vi "HXG2-Main_R2.vi"() -> ()   [LabVIEW 2012]
uses:
  Controls/UI/HXG2_NumDisplayOnlyLarge.ctl
  Controls/UI/HXG2_UI_ControlSetGly.ctl
  Controls/UI/HXG2_UI_ControlSetAir.ctl
  Controls/UI/HXG2_AirENfanRect.ctl
  Controls/UI/HXG2_GlyENfanRect.ctl
  Controls/UI/HXG2_NumDisplayLarge.ctl
  Controls/HXG2_AlarmCluster.ctl
  Controls/UI/HXG2_LED.ctl
  Controls/HXG2_DAQLOOPctrl.ctl
  Modules/Programmer/Data Types/Programmer State.ctl
  Controls/UI/HXG2_NumDisplayOnlySmall.ctl
  Controls/UI/HXG2_MainStateCtrl.ctl
  Controls/UI/HXG2_GralTubeData.ctl
  Controls/UI/HXG2_FinData.ctl
  PID/HXG2_Horizontal PID Control.ctl
  PID/HXG2_Horizontal Reset Control.ctl
  <vilib>/Utility/error.llb/DialogType.ctl
  Modules/Error_Handler/HXG2-Error_Module.ctl
  Modules/Stop/HXG2stop.ctl
  Modules/EnableAirGly/HXG2enable.ctl
  Modules/Timers/HXG2_BlowerPumpl.ctl
  Modules/PID/HXG2pid.ctl
  Modules/Graph_Scales/HXG2_GraphSelections.ctl
  Controls/HXG2_BooleanSelections.ctl
  Modules/BooleanSelections/HXG2boolselec.ctl
  Modules/Save/HXG2save.ctl
  Modules/Save/HXG2saveTimer.ctl
  Modules/AIR-GLY_Clusters/HXG2airglyCluster.ctl
  Controls/HXG2_PIDon-off.ctl
  Modules/DataTransfer/HXG2DataTrans.ctl
  Controls/HXG2_DigitalIn.ctl
  Modules/Programmer/HXG2programmer.ctl
  Modules/Programmer/HXG2programmerUserSelections.ctl
  Modules/Programmer/Data Types/Programmer Execution States.ctl
  Modules/Programmer/HXG2_ProgRefs.ctl
  CondensingVIs/PIDCtrl/HXG2_References.ctl
  <vilib>/Utility/miscctls.llb/LVRowAndColumnTypeDef.ctl
  Controls/HXG2_PIDCluster.ctl
  Controls/HXG2_Aircool-Cascade.ctl
  Controls/HXG2_LiqHeat-Cascade.ctl
  Modules/DAQ/HXG2daq.ctl
  <vilib>/DAQmx/write.llb/DAQmx Write (Digital 1D Bool NChan 1Samp 1Line).vi
panel:
  out "MAIN":bool
  out "DAQ":bool
  in  "HX ID":string="Description #" caption="CHANGE ID OR CLICK TO ACCEPT"
  out "Clear Alarms":bool
  in  "stop":bool
  in  "Master RUN":bool
  out "Main Ctrl":T1
  out "DAQ Control":T2
  out "Event":i32
  out "Main":i32
  out "daq":i32
  in  "Alarm Set Button":bool
  out "error out":errorcluster
  out "Alarm Cluster":T3
  in  "error in (no error)":errorcluster
  out "Programmer":bool
  in  "Tab Control":T5(tab)
  out "dP Inlet":dbl(knob) scale=-10.0..20.0
  out "Pump Pressure (150psi max)":dbl(knob) scale=14.56..50.0
  out "Re Number":dbl format="%#.0f"
  in  "Select Tube OD":u16(ring) items=["3/8\"", "5/16\"", "1/4\"", "3/16\"", "custom"]
  in  "Tube ID (in)":dbl=1.0 min=0.1 max=1.0 format="%#.2f"
  out "Min ACFM 2":dbl format="%#.2f"
  out "Max ACFM 2":dbl format="%#.2f"
  out "HX Pressure In":dbl format="%#.2f psig"
  out "HX dP":dbl format="%#.2f psid"
  out "Pump Pressure":dbl format="%#.2f psig"
  out "Discharge Temp":dbl format="%#.2f °F"
  out "Suction Temp":dbl format="%#.2f °F"
  out "Comp\nSuct SH":dbl format="%#.2f °F"
  out "Comp Suct P psia":dbl(knob) scale=15.0..30.0 scale format="%#.2f"
  in  "Reset Alarm UI":bool
  out "Alarm Present\nLED":bool
  out "Liq Temp °F":T6 min=0.0 max=100.0 format="%#.1f"
  in  "LT PID":bool
  in  "LF PID":bool
  in  "Liq Cluster":T7={"Liq FLOW %"=0.0, "Liq TEMP % "=50.0, "Mdot lbm/hr"=0.0, "TLiq °F"=70.0} caption="Gly Cluster" {"Liq TEMP %" min=0.0 max=100.0 step=1.0 format="%#.1f"; "Liq FLOW %" min=0.0 max=100.0 step=1.0 format="%#.1f"; "TLiq °F" min=40.0 max=180.0 step=1.0 format="%#.1f"; "Mdot lbm/hr" min=0.0 max=1000.0 step=1.0 format="%#.1f"}
  in  "AT PID":bool
  in  "Air Cluster":T8={"Air FLOW %"=30.0, "Air TEMP % "=50.0, "CFMs"=30.0, "Tair  °F"=70.0} {"Air TEMP %" min=0.0 max=100.0 step=1.0 format="%#.1f"; "Air FLOW %" min=0.0 max=100.0 step=1.0 format="%#.1f"; "Tair  °F" min=-5.0 max=100.0 step=1.0 format="%#.1f"; "CFMs" min=0.0 max=200.0 step=1.0 format="%#.1f"}
  in  "Air EN":T9
  out "Air Flow ACFM":T6 min=0.0 max=100.0 format="%#.1f"
  out "Air Temp °F":T6 min=0.0 max=100.0 format="%#.1f"
  in  "LIQ EN":T10
  out "Liq Flow lbm/hr":T11 format="%#.1f"
  in  "Capture Data":bool
  out "Interval Ind":dbl format="%<%H:%M:%S>t"
  out "Duration Ind":dbl format="%<%H:%M:%S>t"
  in  "Duration Ctrl":dbl=15.0 format="%#.1f min"
  in  "Interval Ctrl":dbl=2.0 format="%#.1f s"
  out "File Name":string="Test.tdms"
  out "saving...":bool
  in  "+10":bool
  in  "-10":bool
  in  "Test Point":i32
  in  "AF PID":bool
  out "Pump Pin (psia)":dbl format="%#.2f"
  out "Pump Pout (psia)":dbl format="%#.2f"
  out "UUT dP 0-1.0":dbl format="%.2f inWC"
  out "Liq Htr Well":dbl format="%#.3f °F"
  out "dT Air":dbl format="%#.3f °F"
  out "dT Liq":dbl format="%#.3f °F"
  in  "Sensor":bool
  out "Nozzle dP 2.5inWC":dbl format="%#.3f"
  out "%Bal":string
  out "Max ACFM":dbl format="%#.2f"
  out "Min ACFM":dbl format="%#.2f"
  in  "1\"":bool
  in  "1.25\"":bool
  in  "0.75\"":bool
  in  "1.5\"":bool
  out "Liq q W":dbl format="%#.2f"
  out "Air q W":dbl format="%#.3g"
  out "% Balance":dbl format="%#.1f%"
  out "Air q BTU/hr":dbl format="%#.3g"
  out "Liq q BTU/hr":dbl format="%#.2f"
  out "GlyFlow lbm/hr":dbl format="%#.2f lbm/hr"
  out "LiqCp BTU/lb°F":dbl format="%#.2f"
  out "LiqRho lb/ft³":dbl format="%#.2f"
  out "AirFlow ACFM":dbl format="%#.2f"
  out "AirFlow SCFM":dbl format="%#.2f"
  out "AirCp BTU/lb°F":dbl format="%#.4f"
  out "AirRho lb/ft³":dbl format="%#.4f"
  out "Nozzle °F":dbl format="%#.2f"
  out "UUT °F":dbl format="%#.2f"
  out "Nozzle %RH":dbl format="%#.2f"
  out "UUT %RH":dbl format="%#.2f"
  out "Nozzle dP 5inWC":dbl format="%#.3f"
  out "UUT dP 0-0.1":dbl format="%.3f inWC"
  out "Baro psia":dbl format="%#.2f"
  out "LiqOut Avg °F":dbl format="%#.2f"
  out "LiqIn Avg °F":dbl format="%#.2f"
  out "AirOut Avg °F":dbl format="%#.2f"
  out "AirIn Avg °F":dbl format="%#.2f"
  out "AirOut 8":dbl format="%#.2f"
  out "AirOut 7":dbl format="%#.2f"
  out "AirOut 6":dbl format="%#.2f"
  out "AirOut 4":dbl format="%#.2f"
  out "AirOut 3":dbl format="%#.2f"
  out "AirOut 2":dbl format="%#.2f"
  out "AirOut 1":dbl format="%#.2f"
  in  "AirOut 1 °F":bool
  in  "AirOut 2 °F":bool
  in  "AirOut 3 °F":bool
  in  "AirOut 4 °F":bool
  in  "AirOut 5 °F":bool
  in  "AirOut 6 °F":bool
  in  "AirOut 7 °F":bool
  in  "AirOut 8 °F":bool
  out "AirOut 5":dbl format="%#.2f"
  out "AirIn 4":dbl format="%#.2f"
  out "AirIn 3":dbl format="%#.2f"
  out "AirIn 2":dbl format="%#.2f"
  out "AirIn 1":dbl format="%#.2f"
  in  "AirIn 1 °F":bool
  in  "AirIn 2 °F":bool
  in  "AirIn 3 °F":bool
  in  "AirIn 4 °F":bool
  out "GlyOut 2":dbl format="%#.2f"
  out "GlyOut 1":dbl format="%#.2f"
  in  "LiqOut 1 °F":bool
  in  "LiqOut 2 °F":bool
  out "GlyIn 2":dbl format="%#.2f"
  out "GlyIn 1":dbl format="%#.2f"
  in  "LiqIn 1 °F":bool
  in  "LiqIn 2 °F":bool
  in  "SchedSelect":enum16{"Schedule 1", "Schedule 2", "Schedule 3"}(ring)
  in  "Set Prof 1":bool
  out "Liq Temp":dbl=100.0 format="%#.1f °F"
  out "Mass flow":dbl=100.0 format="%#.1f lbm/hr"
  out "Air Temp":dbl=100.0 format="%#.1f °F"
  out "Air flow":dbl=100.0 format="%#.1f CFM"
  in  "Apply Scales":bool
  in  "Plot Selection":u16[](array[ring]) items=["Liq In Avg", "Liq In 1", "Liq In 2", "Liq Out Avg", "Liq Out 1", "Liq Out 2", "Fltrd Mdot", "Liq Mdot", "Pump 0-250psia", "Pump dP 0-25psid", "UUT 0-100psid", "UUT 0-95psig", "Air In Avg", "Air In 1", "Air In 2", "Air In 3", "Air In 4", "Air Out Avg", "Air Out 1", "Air Out 2", "Air Out 3", "Air Out 4", "Air Out 5", "Air Out 6", "Air Out 7", "Air Out 8", "CFM Nozzle", "CFM HX", "UUT 0-0.1inWC x100", "UUT 0-1inWC x100", "Nozzle 0-5inWC x100", "Nozzle 0-2.5inWC x100", "Pbaro [psia]", "Liq Q (BTU/hr)", "Liq Q (W)", "Air Q (BTU/hr)", "Air Q (W)", "SH (°F)", "SH multiplier", "%Energy Bal", "Liq Re", "AF Ctl Out", "AC Ctl Out", "AH Ctl Out", "LF Ctl Out", "LC Ctl Out", "LH Ctl Out", "Box Btm In (9)", "Box Btm Out (10)", "Box Rt In (11)", "Box Rt Frt (12) ", "Box Top In(13)", "Box Top Out(14)", "Box Lt In (15)", "Box Lt Out (16)", "Evap TR", "Evap TL", "Evap BR", "Evap BL", "Htr Rt", "Htr Top", "Htr Lt", "Htr Btm", "WaterTank"]
  in  "Plot Axis":u32[](array[ring]) items=["1", "2", "3"]
  out "Waveform Chart Out":waveform(dbl)[](graph)
  in  "Max 1":dbl=100.0
  in  "Min 1":dbl
  in  "Max 2":dbl=100.0
  in  "Min 2":dbl
  in  "Max 3":dbl=100.0
  in  "Min 3":dbl
  in  "x-axis length (min)":dbl=1.0
  out "% Balance":dbl format="%#.1f%"
  out "%Bal2":string
  in  "Set Prof 2":bool
  in  "Set Prof 3":bool
  in  "Default":bool
  in  "PID Setup Array":T12
  in  "PID Select":T13(ring)
  in  "Reset PIDs":T14
  in  "Fan TR":bool
  in  "Fan TL":bool
  in  "Fan BL":bool
  in  "Fan BR":bool
  out "Timer":dbl format="%<%H:%M:%S%1u>t"
  in  "HX ID (in)":dbl
  in  "Target Re":dbl
  in  "Liq Tin (°F)":dbl
  out "mdot (lbm/hr)":dbl
  out "mu (lbm/ft*s)":dbl
  out "Cp (BTU/lbm°F)":dbl
  out "Density (lbm/ft³)":dbl
  in  "Repeat Execution:":i32
  in  "Done Stop":bool=TRUE
  in  "Run Programmer":bool
  in  "Load Profile":bool
  in  "Save Profile":bool
  in  "Table":string[][](table) caption="StartProf.prof"
  out "Current Step":i32
  out "Programmer State":T15
  out "AirFlow Stable":bool
  out "AirTemp Stable":bool
  out "LiqFlow Stable":bool
  out "LiqTemp Stable":bool
  out "CFM SP":T16 min=0.0 max=100.0 format="%#.1f"
  out "Tair SP °F":T16 min=0.0 max=100.0 format="%#.1f"
  out "Liq SP lbm/hr":T16 min=0.0 max=100.0 format="%#.1f"
  out "Tliq SP °F":T16 min=0.0 max=100.0 format="%#.1f"
  out "Tliq  °F":T16 min=0.0 max=100.0 format="%#.1f"
  out "Filtered Mdot lbm/hr":T16 min=0.0 max=100.0 format="%#.1f"
  out "Tair  °F":T16 min=0.0 max=100.0 format="%#.1f"
  out "CFM":T16 min=0.0 max=100.0 format="%#.1f"
  out "Ring Text.Text":string
  out "UUTIn 5":dbl format="%#.1f °F"
  out "UUTIn 6":dbl format="%#.1f °F"
  out "UUTIn 7":dbl format="%#.1f °F"
  out "UUTIn 8":dbl format="%#.1f °F"
  out "UUTIn 1":dbl format="%#.1f °F"
  out "UUTIn 2":dbl format="%#.1f °F"
  out "UUTIn 3":dbl format="%#.1f °F"
  out "UUTIn 4":dbl format="%#.1f °F"
  in  "TC 8":string
  in  "TC 7":string
  in  "TC 6":string
  in  "TC 5":string
  in  "TC 4":string
  in  "TC 3":string
  in  "TC 2":string
  in  "TC 1":string
  in  "Prof 3":u16[](array[ring]) items=["Liq In Avg", "Liq In 1", "Liq In 2", "Liq Out Avg", "Liq Out 1", "Liq Out 2", "Fltrd Mdot", "Liq Mdot", "Pump 0-250psia", "Pump dP 0-25psid", "UUT 0-100psid", "UUT 0-95psig", "Air In Avg", "Air In 1", "Air In 2", "Air In 3", "Air In 4", "Air Out Avg", "Air Out 1", "Air Out 2", "Air Out 3", "Air Out 4", "Air Out 5", "Air Out 6", "Air Out 7", "Air Out 8", "CFM Nozzle", "CFM HX", "UUT 0-0.1inWC x100", "UUT 0-1inWC x100", "Nozzle 0-5inWC x100", "Nozzle 0-2.5inWC x100", "Pbaro [psia]", "Liq Q (BTU/hr)", "Liq Q (W)", "Air Q (BTU/hr)", "Air Q (W)", "SH (°F)", "SH multiplier", "%Energy Bal", "Liq Re", "AF Ctl Out", "AC Ctl Out", "AH Ctl Out", "LF Ctl Out", "LC Ctl Out", "LH Ctl Out", "Box Btm In (9)", "Box Btm Out (10)", "Box Rt In (11)", "Box Rt Frt (12) ", "Box Top In(13)", "Box Top Out(14)", "Box Lt In (15)", "Box Lt Out (16)", "Evap TR", "Evap TL", "Evap BR", "Evap BL", "Htr Rt", "Htr Top", "Htr Lt", "Htr Btm", "WaterTank"]
  in  "Prof 2":u16[](array[ring]) items=["Liq In Avg", "Liq In 1", "Liq In 2", "Liq Out Avg", "Liq Out 1", "Liq Out 2", "Fltrd Mdot", "Liq Mdot", "Pump 0-250psia", "Pump dP 0-25psid", "UUT 0-100psid", "UUT 0-95psig", "Air In Avg", "Air In 1", "Air In 2", "Air In 3", "Air In 4", "Air Out Avg", "Air Out 1", "Air Out 2", "Air Out 3", "Air Out 4", "Air Out 5", "Air Out 6", "Air Out 7", "Air Out 8", "CFM Nozzle", "CFM HX", "UUT 0-0.1inWC x100", "UUT 0-1inWC x100", "Nozzle 0-5inWC x100", "Nozzle 0-2.5inWC x100", "Pbaro [psia]", "Liq Q (BTU/hr)", "Liq Q (W)", "Air Q (BTU/hr)", "Air Q (W)", "SH (°F)", "SH multiplier", "%Energy Bal", "Liq Re", "AF Ctl Out", "AC Ctl Out", "AH Ctl Out", "LF Ctl Out", "LC Ctl Out", "LH Ctl Out", "Box Btm In (9)", "Box Btm Out (10)", "Box Rt In (11)", "Box Rt Frt (12) ", "Box Top In(13)", "Box Top Out(14)", "Box Lt In (15)", "Box Lt Out (16)", "Evap TR", "Evap TL", "Evap BR", "Evap BL", "Htr Rt", "Htr Top", "Htr Lt", "Htr Btm", "WaterTank"]
  out "UUTIn 15":dbl format="%#.1f °F"
  out "UUTIn 11":dbl format="%#.1f °F"
  out "UUTIn 10":dbl format="%#.1f °F"
  out "UUTIn 9":dbl format="%#.1f °F"
  out "UUTIn 14":dbl format="%#.1f °F"
  out "UUTIn 13":dbl format="%#.1f °F"
  in  "Accuracy (%of flow)":dbl=0.05
  in  "Repeatability (% of flow)":dbl=0.025
  in  "Select Path":path
  in  "Inlet  Uncert (°F)":dbl=0.09
  in  "Outlet  Uncert (°F)":dbl=0.09
  out "Liquid Power Uncertainty":T17 {"% error T" format="%#.3f"; "% error Power" format="%#.3f"; "% error Mdot" format="%#.3f"; "Power Uncert (BTU/hr)" format="%#.3f"; "Power Uncert (W)" format="%#.3f"}
  out "UUTIn 12":dbl format="%#.1f °F"
  out "UUTIn 16":dbl format="%#.1f °F"
  in  "Prof 1":u16[](array[ring]) items=["Liq In Avg", "Liq In 1", "Liq In 2", "Liq Out Avg", "Liq Out 1", "Liq Out 2", "Fltrd Mdot", "Liq Mdot", "Pump 0-250psia", "Pump dP 0-25psid", "UUT 0-100psid", "UUT 0-95psig", "Air In Avg", "Air In 1", "Air In 2", "Air In 3", "Air In 4", "Air Out Avg", "Air Out 1", "Air Out 2", "Air Out 3", "Air Out 4", "Air Out 5", "Air Out 6", "Air Out 7", "Air Out 8", "CFM Nozzle", "CFM HX", "UUT 0-0.1inWC x100", "UUT 0-1inWC x100", "Nozzle 0-5inWC x100", "Nozzle 0-2.5inWC x100", "Pbaro [psia]", "Liq Q (BTU/hr)", "Liq Q (W)", "Air Q (BTU/hr)", "Air Q (W)", "SH (°F)", "SH multiplier", "%Energy Bal", "Liq Re", "AF Ctl Out", "AC Ctl Out", "AH Ctl Out", "LF Ctl Out", "LC Ctl Out", "LH Ctl Out", "Box Btm In (9)", "Box Btm Out (10)", "Box Rt In (11)", "Box Rt Frt (12) ", "Box Top In(13)", "Box Top Out(14)", "Box Lt In (15)", "Box Lt Out (16)", "Evap TR", "Evap TL", "Evap BR", "Evap BL", "Htr Rt", "Htr Top", "Htr Lt", "Htr Btm", "WaterTank"]
  out "EvapAvg":dbl format="%#.1f °F"
  out "HtrAvg":dbl format="%#.1f °F"
  in  "AirCool Cascade":T18={"PID gains"={"proportional gain (Kc)"=-1.15, "integral time (Ti, min)"=2.44, "derivative time (Td, min)"=0.0}, "output range"={"output high"=100.0, "output low"=10.0}} {"output range"."output low" format="%.2f"; "output range"."output high" format="%.2f"; "PID gains"."derivative time (Td, min)" format="%.3f"; "PID gains"."integral time (Ti, min)" format="%.3f"; "PID gains"."proportional gain (Kc)" format="%.3f"}
  out "Calc Rho (lbm/ft³)":dbl=65.0 format="%#.5f"
  out "T° @ f/meter":dbl=65.0 format="%#.5f"
  out "Cp (BTU/lbm °F)":dbl=65.0 format="%#.4f"
  out "Viscosity (lbm/ft s)":dbl=65.0 format="%#.5f"
  in  "LiqHeat Cascade":T18={"PID gains"={"proportional gain (Kc)"=3.54, "integral time (Ti, min)"=46.25, "derivative time (Td, min)"=0.0}, "output range"={"output high"=100.0, "output low"=0.0}} {"output range"."output low" format="%.2f"; "output range"."output high" format="%.2f"; "PID gains"."derivative time (Td, min)" format="%.3f"; "PID gains"."integral time (Ti, min)" format="%.3f"; "PID gains"."proportional gain (Kc)" format="%.3f"}
  in  "CoilData Tabs":enum32{"General Data", "Fin Data"}(tab)
  in  "General_Tube data":T19 {"Tube vertical spacing (Sf)" format="%#.3f in"; "Tube horizontal spacing (Sr)" format="%#.3f in"; "Tube ID" format="%#.3f in"; "Tube thickness" format="%#.3f in"; "Tube OD" format="%#.3f in"; "Tube test Length (tL)" format="%#.3f in"}
  in  "Fin Data":T20 {"Ext collar length" format="%#.3f in"; "Tubes per plate" format="%#.3f"; "Wire Diameter" format="%#.3f in"; "Fin stretch ratio" format="%#.3f %"; "Fin thickness" format="%#.3f in"; "Fin Width" format="%#.3f in"; "Fin OD" format="%#.3f in"; "Fin contact resistance" format="%#.3f ft² hr °F/BTU"; "Fins per inch (FPI)" format="%#.3f"}
  # "10min"
  # "psia"
  # "dP"
  # "RESET"
  # "On 2.5inWC"
  # "Off 5inWC"
  # "NOZZLES"
  # "TARGETS"
  # "times"
  # "RTDs"
  # "Mass Flow"
  # "GRAPH PROFILES"
  # "1"
  # "2"
  # "3"
  # "Heater Outlet\n(Air into screen)"
  # "Evaporator Outlet\n   (Air into screen)"
  # "Coil Physical Data"
  # "Spine Fin"
  # "Wire Fin"
  # "Plate Fin"
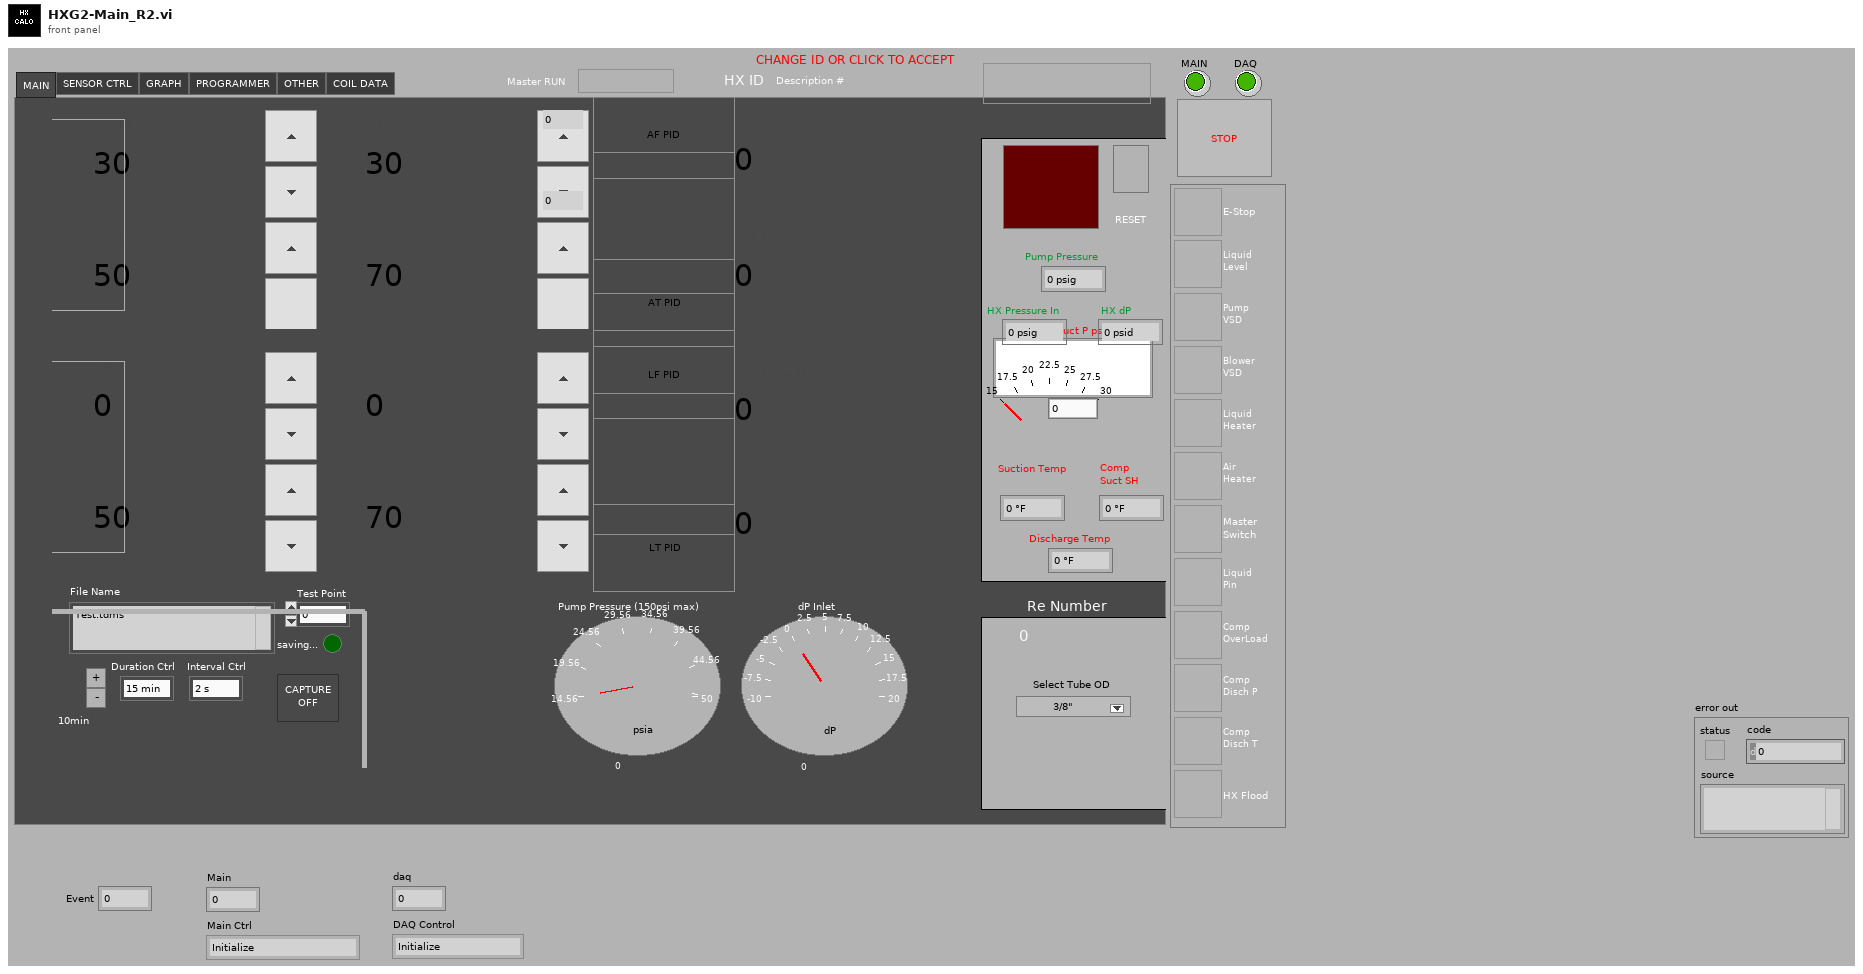
[diagram p1: front panel]
types:
  T1 = typedef "HXG2_MainStateCtrl.ctl" = enum16{"Initialize", "Initialize UI", "DAQ", "Process", "Control", "Write", "Save", "Print", "Graph", "Sequencer", "ERROR", "Exit"}
  T2 = typedef "HXG2_DAQLOOPctrl.ctl" = enum16{"Initialize", "DAQ", "Stop"}
  T3 = typedef "HXG2_AlarmCluster.ctl" = cluster{"E-Stop":T4, "Liquid\nLevel":T4, "Pump\nVSD":T4, "Blower\nVSD":T4, "Liquid\nHeater":T4, "Air\nHeater":T4, "Master\nSwitch":T4, "Liquid\nPin":T4, "Comp\nOverLoad":T4, "Comp\nDisch P":T4, "Comp \nDisch T":T4, "HX Flood":T4}
  T4 = typedef "HXG2_LED.ctl" = bool
  T5 = enum32{"MAIN", "SENSOR CTRL", "GRAPH", "PROGRAMMER", "OTHER", "COIL DATA"}
  T6 = typedef "HXG2_NumDisplayOnlyLarge.ctl" = dbl
  T7 = typedef "HXG2_UI_ControlSetGly.ctl" = cluster{"Liq FLOW %":dbl, "Liq TEMP % ":dbl, "Mdot lbm/hr":dbl, "TLiq °F":dbl}
  T8 = typedef "HXG2_UI_ControlSetAir.ctl" = cluster{"Air FLOW %":dbl, "Air TEMP % ":dbl, "CFMs":dbl, "Tair  °F":dbl}
  T9 = typedef "HXG2_AirENfanRect.ctl" = bool
  T10 = typedef "HXG2_GlyENfanRect.ctl" = bool
  T11 = typedef "HXG2_NumDisplayLarge.ctl" = dbl
  T12 = typedef "HXG2_Horizontal PID Control.ctl" = cluster{"GainsArray":cluster{"Gains 2":cluster{"P":dbl, "I, sec":dbl, "D, sec":dbl}, "Max\nPV":dbl}[], "UL-LL Array":cluster{"UL":dbl, "LL  ":dbl}[]}[]
  T13 = enum16{"AIRFLOW", "AIRCOOL", "AIRHEAT", "LIQFLOW", "LIQCOOL", "LIQHEAT"}
  T14 = typedef "HXG2_Horizontal Reset Control.ctl" = cluster{"AF":bool, "AC":bool, "AH":bool, "LF":bool, "LC":bool, "LH":bool}
  T15 = typedef "Programmer State.ctl" = enum16{"Prepare Next Test Step", "Stopped", "Running", "Stabilizing"}
  T16 = typedef "HXG2_NumDisplayOnlySmall.ctl" = dbl
  T17 = cluster{"Power (BTU/hr)":dbl, "Power Uncert (W)":dbl, "Power Uncert (BTU/hr)":dbl, "% error Mdot":dbl, "% error Power":dbl, "% error T":dbl}
  T18 = cluster{"PID gains":cluster{"proportional gain (Kc)":dbl, "integral time (Ti, min)":dbl, "derivative time (Td, min)":dbl}, "output range":cluster{"output high":dbl, "output low":dbl}}
  T19 = typedef "HXG2_GralTubeData.ctl" = cluster{"Date":string, "Mfr. Name":string, "Tested by":string, "Adv Sys Test#":string, "Model Size/Type":string, "Coil Type":string, "Air flow Direction":enum32{"Radio Selection 1", "Radio Selection 2", "Radio Selection 3"}, "Coil Face Orientation":enum32{"Radio Selection 1", "Radio Selection 2", "Radio Selection 3"}, "Tube Orientation":enum32{"Radio Selection 1", "Radio Selection 2", "Radio Selection 3"}, "Tubes per Bank":dbl, "Number of tube banks":dbl, "Tube test Length (tL)":dbl, "Tube OD":dbl, "Tube thickness":dbl, "Tube ID":dbl, "Tube horizontal spacing (Sr)":dbl, "Tube vertical spacing (Sf)":dbl}
  T20 = typedef "HXG2_FinData.ctl" = cluster{"Fins per inch (FPI)":dbl, "Fin contact resistance":dbl, "Fin OD":dbl, "Fin Width":dbl, "Fin thickness":dbl, "Fin stretch ratio":dbl, "Wire Diameter":dbl, "Tubes per plate":dbl, "Ext collar length":dbl}
  T21 = typedef "HXG2-Error_Module.ctl" = enum16{"Initialize", "Handle", "Report"}
  T22 = typedef "DialogType.ctl" = u16
  T23 = typedef "HXG2stop.ctl" = enum16{"Write", "Pass"}
  T24 = typedef "HXG2enable.ctl" = enum16{"Write Refs", "Write", "Pass"}
  T25 = typedef "HXG2_BlowerPumpl.ctl" = enum16{"Stop", "Start", "Check Time"}
  T26 = typedef "HXG2pid.ctl" = enum16{"Write PID Efforts", "Write PID On-Off", "Pass", "Write PID Refs", "Write PID Gains", "Wrt PID Resets"}
  T27 = typedef "HXG2_GraphSelections.ctl" = enum16{"Load From File", "Plot Selection In", "Plot Axis In", "Graph Scales In", "Apply Scales", "Out"}
  T28 = typedef "HXG2boolselec.ctl" = enum16{"Write", "Pass"}
  T29 = typedef "HXG2_BooleanSelections.ctl" = cluster{"Bool":cluster{"Use GlyIn 1":bool, "Use GlyIn 2":bool, "Use GlyOut 1":bool, "Use GlyOut 2":bool, "Use AirIn 1":bool, "Use AirIn 2":bool, "Use AirIn 3":bool, "Use AirIn 4":bool, "Use AirOut 1":bool, "Use AirOut 2":bool, "Use AirOut 3":bool, "Use AirOut 4":bool, "Use AirOut 5":bool, "Use AirOut 6":bool, "Use AirOut 7":bool, "Use AirOut 8":bool, "0.75in Nozzle":bool, "1.00in Nozzle":bool, "1.25in Nozzle":bool, "1.5in Nozzle":bool, "On 2.5inWC/Off 5inWC":bool, "Fan TR":bool, "Fan TL":bool, "Fan BR":bool, "Fan BL":bool}, "Other":cluster{"Tube ID":dbl}}
  T30 = typedef "HXG2save.ctl" = enum16{"Write", "Pass", "Initialize", "Kill"}
  T31 = typedef "HXG2saveTimer.ctl" = enum16{"EvntStrtDurtn", "EvntStrtInterv", "Stop", "Check", "RegStrtInterv", "Add10Durtn", "Take10Durtn"}
  T32 = typedef "HXG2airglyCluster.ctl" = enum16{"Write", "Pass"}
  T33 = typedef "HXG2_PIDon-off.ctl" = cluster{"AF PID":bool, "AT PID":bool, "LF PID":bool, "LT PID":bool}
  T34 = typedef "HXG2_DigitalIn.ctl" = cluster{"All Digital IN":cluster{"LiqNotlow":bool, "LiqHtrNotOverTemp":bool, "AirHtrNotOverTemp":bool, "BlowerVFD-On":bool, "PumpVFD-On":bool, "CompNotOverloaded":bool, "CompNotOverPdisch":bool, "EMOcleared":bool, "EMOreset":bool, "Master Power Switch":bool, "HX Flood":bool}}
  T35 = typedef "HXG2DataTrans.ctl" = enum16{"Write", "Pass"}
  T36 = typedef "HXG2programmer.ctl" = enum16{"Write Refs", "Write Selec", "Write All", "Pass All", "React", "Write Path"}
  T37 = typedef "HXG2programmerUserSelections.ctl" = cluster{"Run Prog":bool, "Done Stop":bool, "Load Profile":bool, "Save Profile":bool, "Repeat Execution:":i32, "Start Programmer":bool, "Stop Programmer":bool}
  T38 = enum8{"Enabled", "Disabled", "Disabled and Grayed Out"}
  T39 = enum16{"AIRFLOW", "AIRCOOL", "AIRHEAT", "LIQFLOW", "LIQCOOL", "LIQHEAT"}[]
  T40 = enum16{"Schedule 1", "Schedule 2", "Schedule 3"}[]
  T41 = typedef "HXG2_PIDctrlsOUT.ctl" = cluster{"Iteration dT (s)":dbl, "af ctrl effort":dbl, "ac ctrl effort":dbl, "ah ctrl effort":dbl, "lf ctrl effort":dbl, "lc ctrl effort":dbl, "lh ctrl effort":dbl}
  T42 = typedef "HXG2_References.ctl" = cluster{"AF PID ON":refnum<vi>, "AT PID ON":refnum<vi>, "LT PID ON":refnum<vi>, "LF PID ON":refnum<vi>, "Reset Ctrls":refnum<vi>[]}
  T43 = typedef "HXG2_ProgRefs.ctl" = cluster{"Prog. Indicator":refnum<vi>, "Table":refnum<vi>, "Save Button":refnum<vi>, "Duration Ctrl":refnum<vi>, "Run Prog":refnum<vi>}
  T44 = typedef "Programmer Execution States.ctl" = enum16{"Register Steps", "Initialize", "Start Test Sequence", "Register Data", "Execute Programmer", "Set Number of Repetitions", "Get Current Step Index", "Get Time Until Step Ends"}
  T45 = typedef "LVRowAndColumnTypeDef.ctl" = cluster{"Row":i32, "Column":i32}
  T46 = typedef "HXG2_PIDCluster.ctl" = cluster{"PIDon-off ":T33, "PID":T12, "Reset PIDs":T14, "AirCool Cascade":T47, "LiqHeat Cascade":T48}
  T47 = typedef "HXG2_Aircool-Cascade.ctl" = cluster{"PID gains":cluster{"proportional gain (Kc)":dbl, "integral time (Ti, min)":dbl, "derivative time (Td, min)":dbl}, "output range":cluster{"output high":dbl, "output low":dbl}}
  T48 = typedef "HXG2_LiqHeat-Cascade.ctl" = cluster{"PID gains":cluster{"proportional gain (Kc)":dbl, "integral time (Ti, min)":dbl, "derivative time (Td, min)":dbl}, "output range":cluster{"output high":dbl, "output low":dbl}}
  T49 = typedef "HXG2daq.ctl" = enum16{"Write", "Pass", "Initialize", "Stop"}
  T50 = typedef "HXG2_AnalogIn.ctl" = cluster{"ANALOG":cluster{"Liq in 1":dbl, "Liq in 2":dbl, "Liq out 1":dbl, "Liq out 2":dbl, "AIR in 1":dbl, "AIR in 2":dbl, "AIR in 3":dbl, "AIR in 4":dbl, "AIR out 1":dbl, "AIR out 2":dbl, "AIR out 3":dbl, "AIR out 4":dbl, "AIR out 5":dbl, "AIR out 6":dbl, "AIR out 7":dbl, "AIR out 8":dbl, "RH in Temp":dbl, "RH in":dbl, "RHout Temp":dbl, "RH out":dbl, "Comp Suct P":dbl, "Pabs nozzle":dbl, "Nozzle dp 0-5":dbl, "UUT dp 0-pt1":dbl, "Nozzle dP 0-2.5":dbl, "Pmp  0-250psia":dbl, "UUT  0-100psid":dbl, "UUT 0-50psia":dbl, "TC in 1":dbl, "TC in 2":dbl, "TC in 3":dbl, "TC in 4":dbl, "TC in 5":dbl, "TC in 6":dbl, "TC in 7":dbl, "TC in 8":dbl, "TC in 9":dbl, "TC in 10":dbl, "TC in 11":dbl, "TC in 12":dbl, "TC in 13":dbl, "TC in 14":dbl, "TC in 15":dbl, "TC in 16":dbl, "Liq Mdot":dbl, "UUT dP 0-1":dbl, "Pump dP 0-25":dbl}, "TCsComp":cluster{"CompSuct °F  ":dbl, "CompDisch °F":dbl, "LiqHtrWell °F":dbl}}
  T51 = cluster{"Excel/Elapsed t":dbl[], "Digital In":T34, "Analog In":T50}
  T52 = typedef "HXG2_AirGly-Cluster.ctl" = cluster{"Air Cluster":T8, "Liq Cluster":T7}
  T53 = cluster{"Airflow (CFM)":dbl, "Air Temp (°F)":dbl, "Glycol Flow (lbm/hr)":dbl, "Glycol Temp(°F)":dbl}
  T54 = typedef "HXG2_Calculated.ctl" = cluster{"Means":cluster{"Liq In Avg":dbl, "Liq Out Avg":dbl, "Air In Avg":dbl, "Air Out Avg":dbl, "%Energy Bal":dbl, "Air Evap Avg":dbl, "Air Htr Avg":dbl, "Air Q low":bool}, "Air":cluster{"Min ACFM":dbl, "Max ACFM":dbl, "CFM nozzle":dbl, "CFM HX":dbl, "Air Q (Btu/hr)":dbl, "Air Q (W)":dbl, "Air Cp (Btu/lb)":dbl, "Air rho (lbm/ft³)":dbl}, "Liq":cluster{"Liq rho (lbm/ft³)":dbl, "Liq Cp (Btu/lb)":dbl, "Liq Q (Btu/hr)":dbl, "Liq Q (W)":dbl, "Liq mu (lbm/ft sec)":dbl, "Liq Conc (%)":dbl, "Tube ID (in)":dbl, "Liq Re":dbl, "Mdot Sensor °F":dbl, "Fltrd Mdot (lbm/hr)":dbl}, "SuperHeat":cluster{"SuperHeat °F":dbl, "Multiplier":dbl}, "dT":cluster{"Air dT °F":dbl, "Liq dT °F":dbl}}
  T55 = typedef "HXG2_MaxConstants.ctl" = cluster{"IN":cluster{"all Digital":refnum<k21>, "all DAQ":refnum<k21>, "Analog 480panel":refnum<k21>, "Freq_Mdot":refnum<k21>}, "OUT":cluster{"DIGITAL":cluster{"all DIGITAL":refnum<k21>}, "allANALOG":cluster{"all ANALOG":refnum<k21>}}}
  T56 = cluster{"Components Stable?[0]":bool, "Components Stable?[1]":bool, "Components Stable?[2]":bool, "Components Stable?[3]":bool}
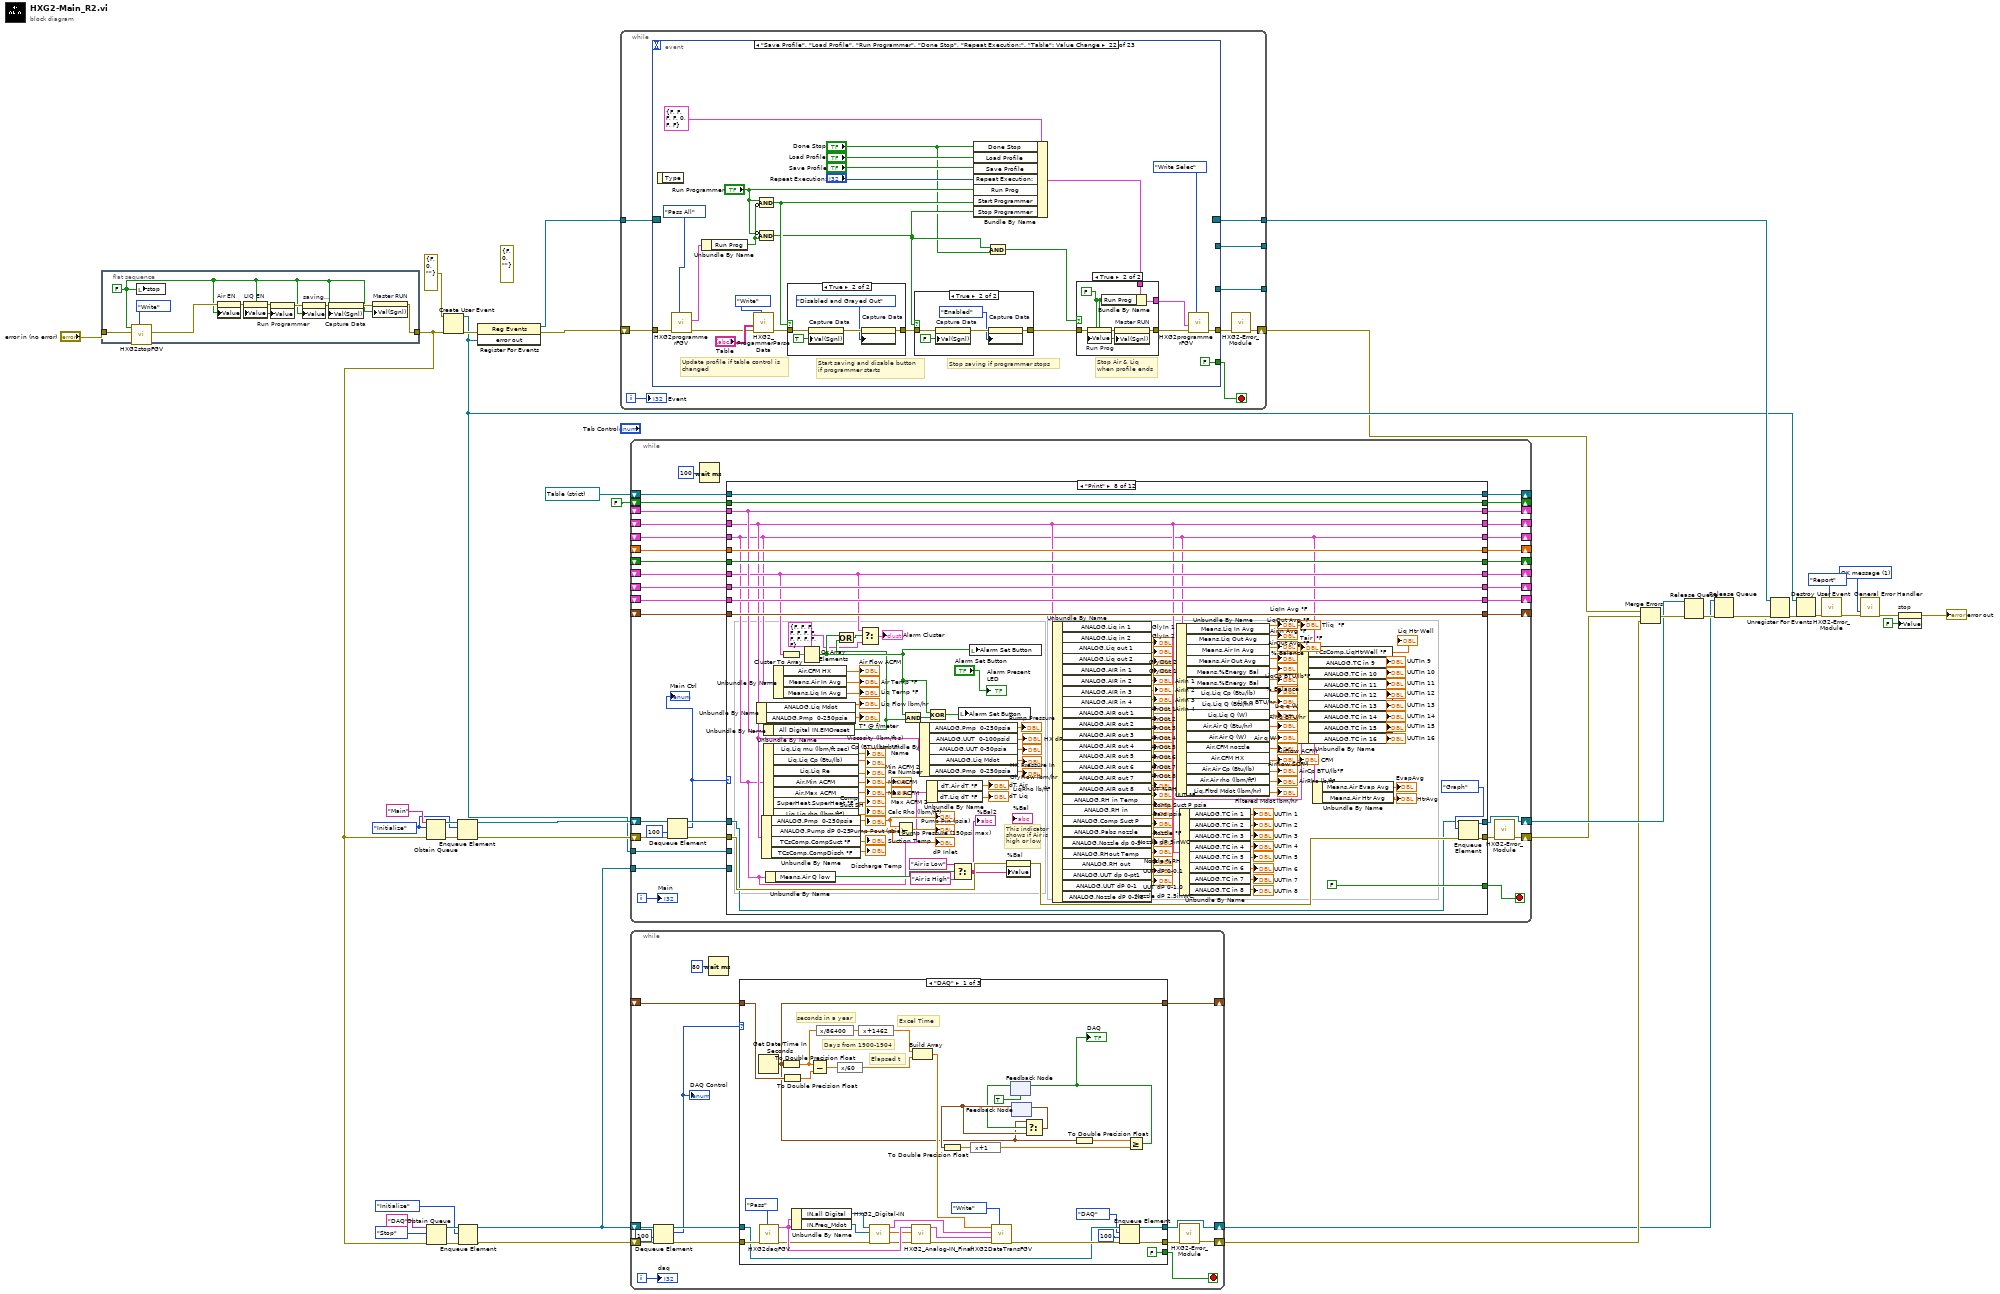
[diagram p0: block diagram]
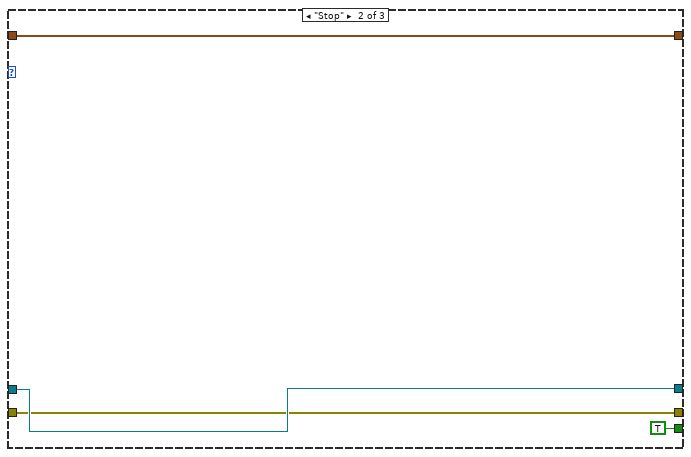
[diagram p2: hidden frame]
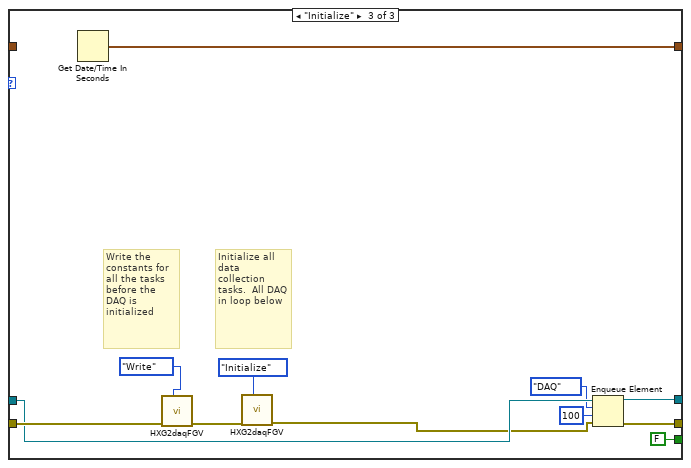
[diagram p3: hidden frame]
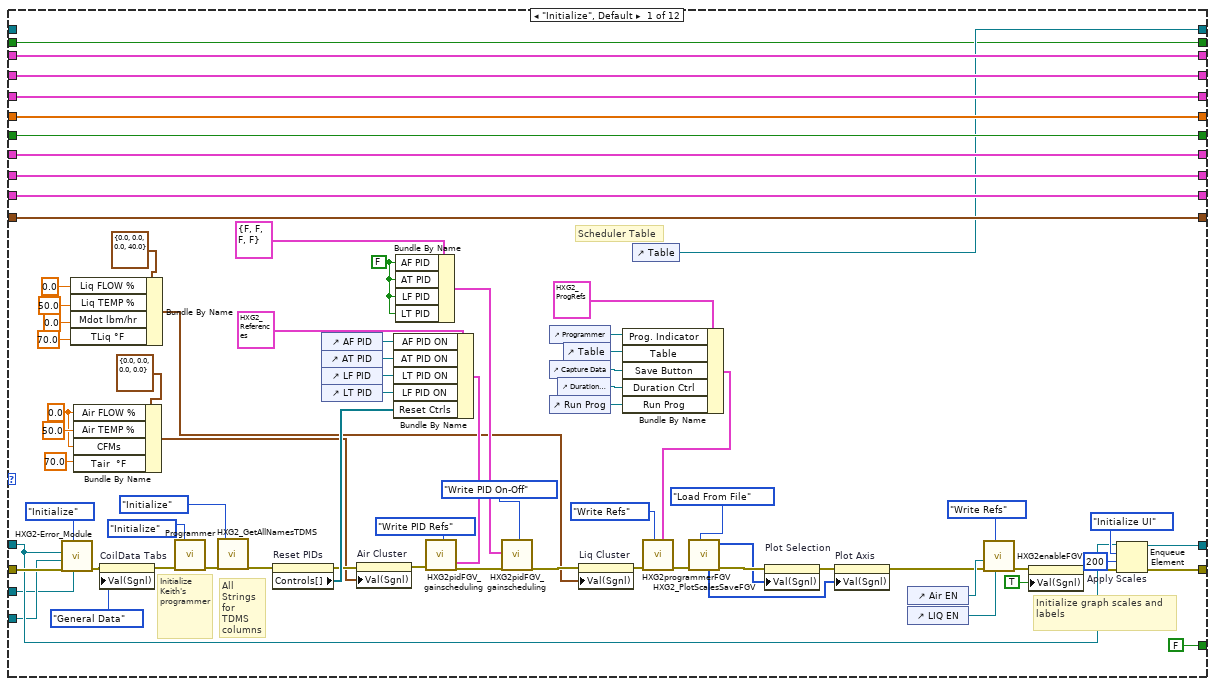
[diagram p4: hidden frame]
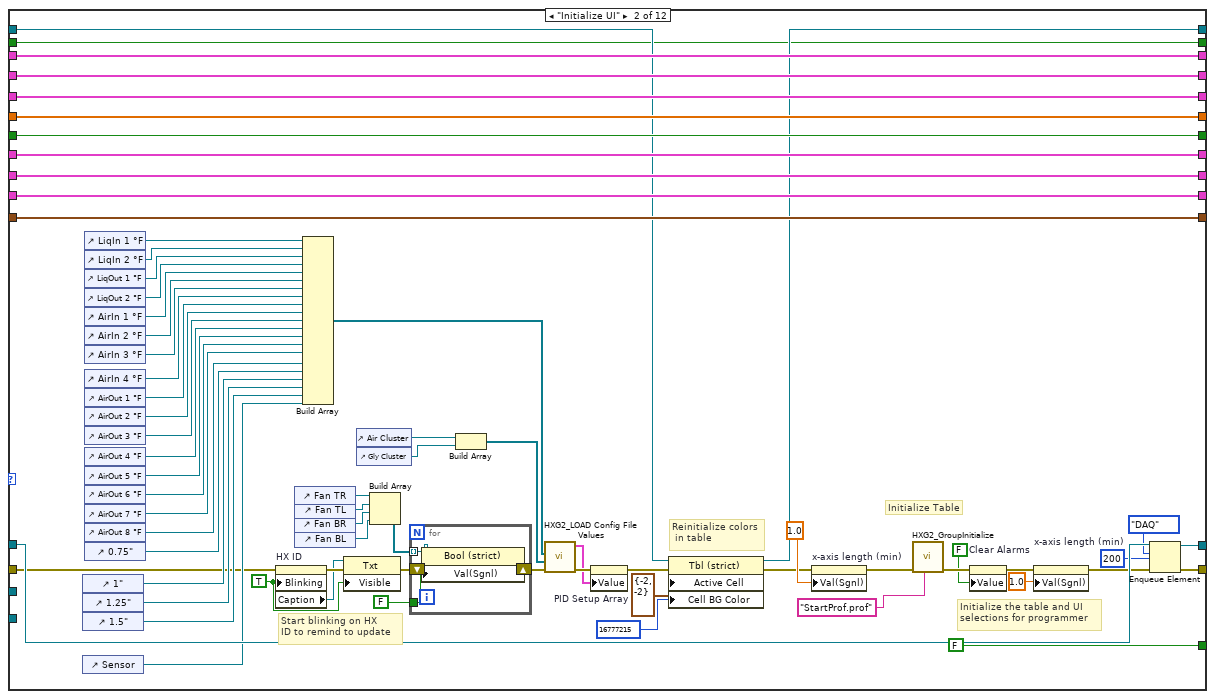
[diagram p5: hidden frame]
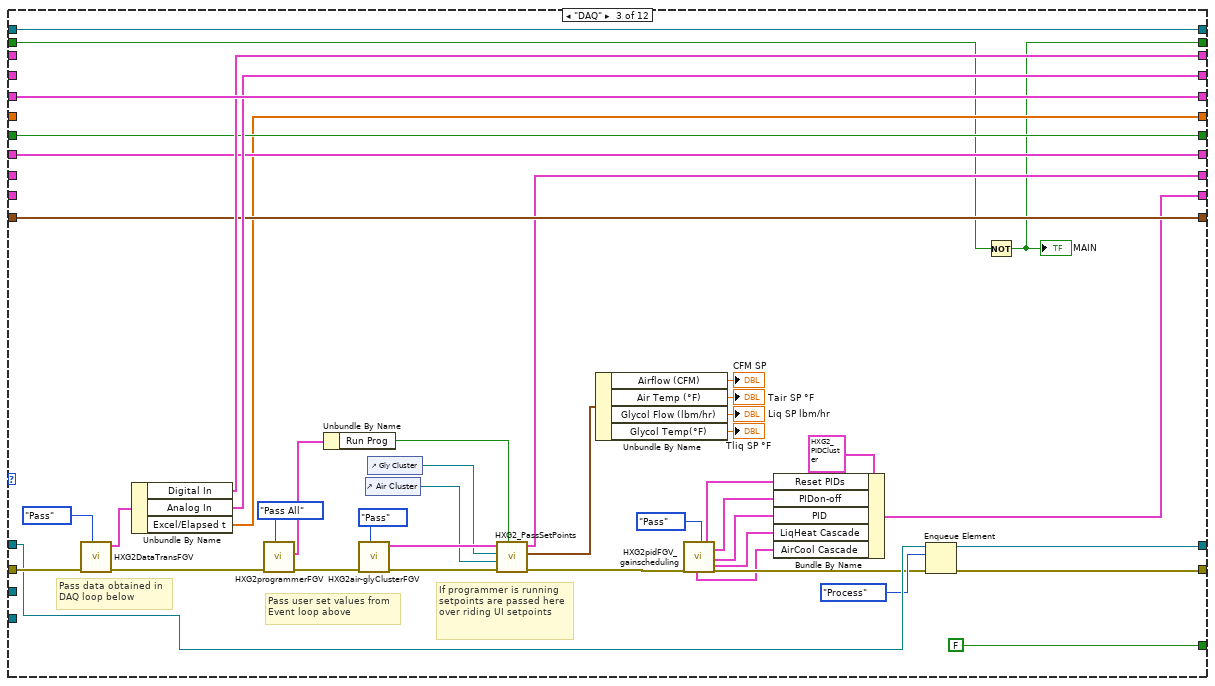
[diagram p6: hidden frame]
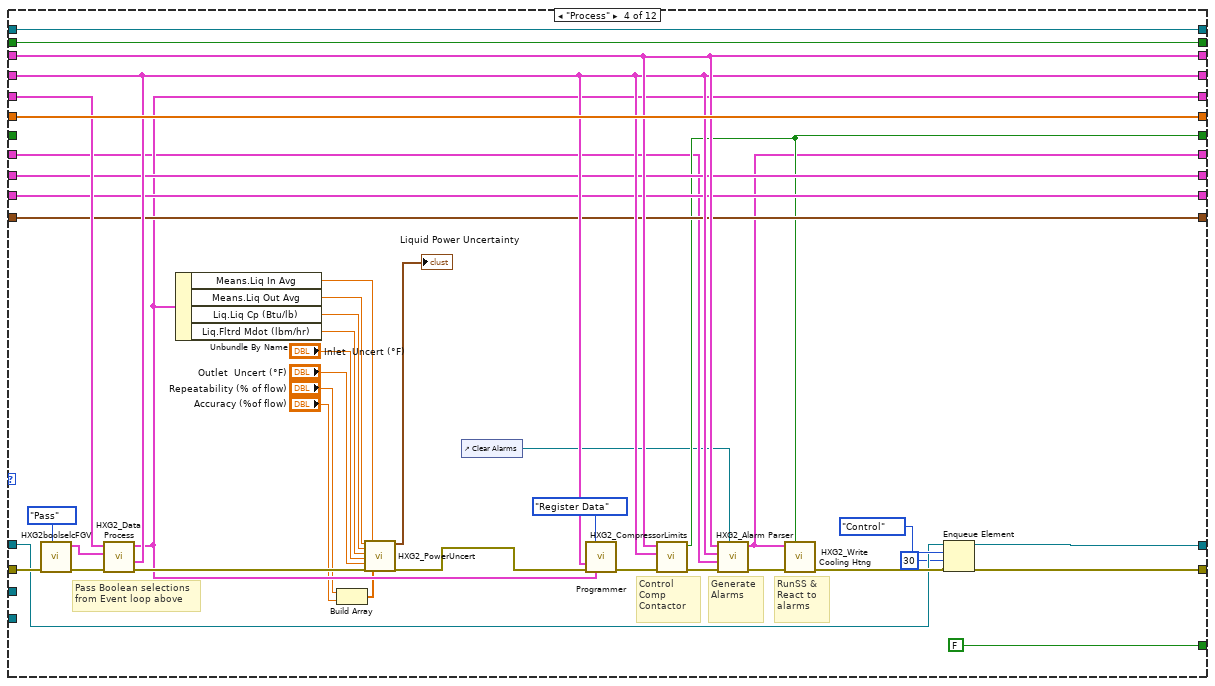
[diagram p7: hidden frame]
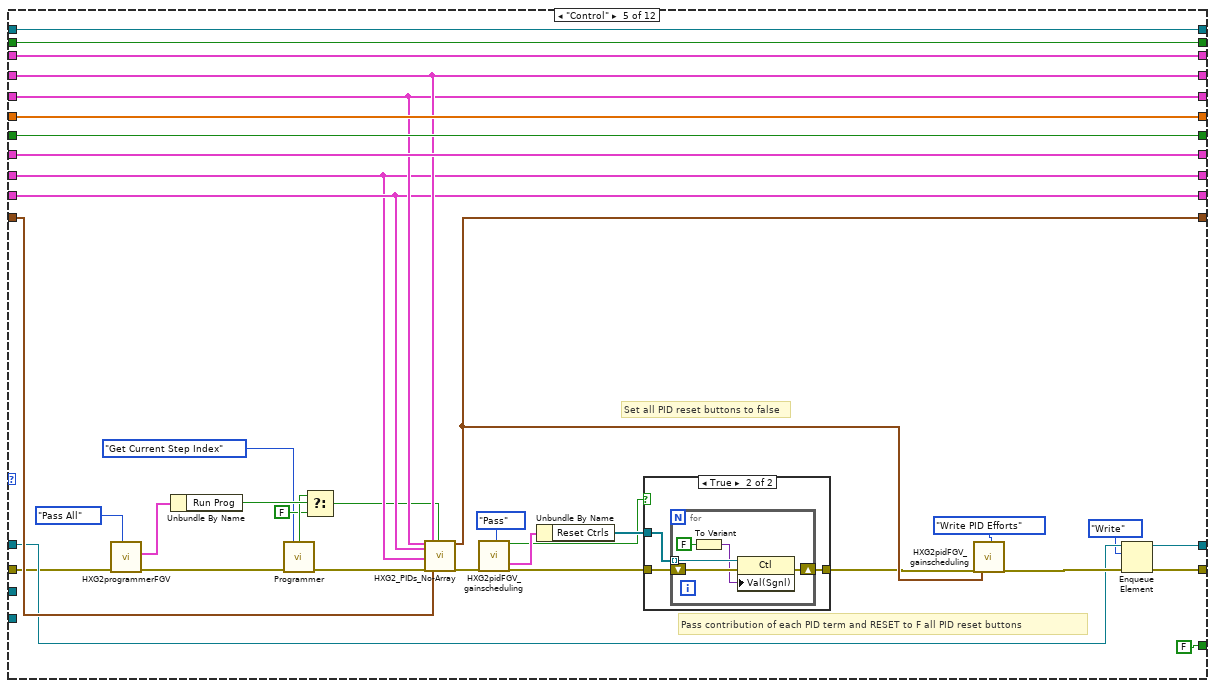
[diagram p8: hidden frame]
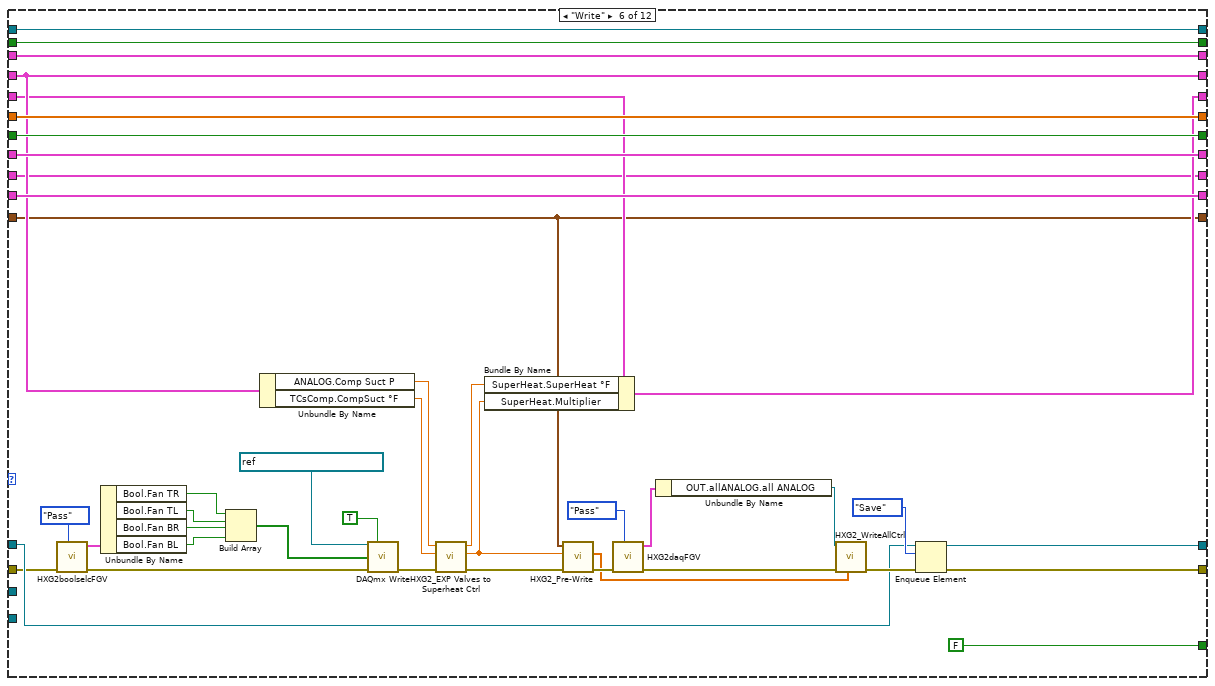
[diagram p10: hidden frame]
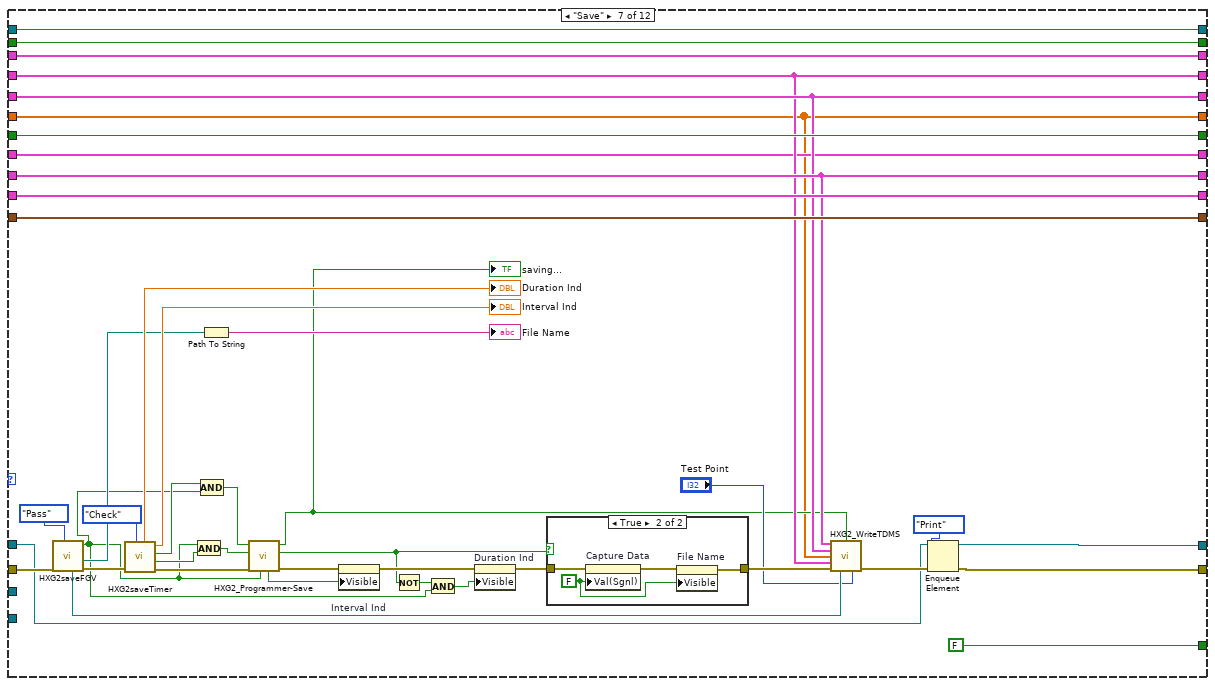
[diagram p11: hidden frame]
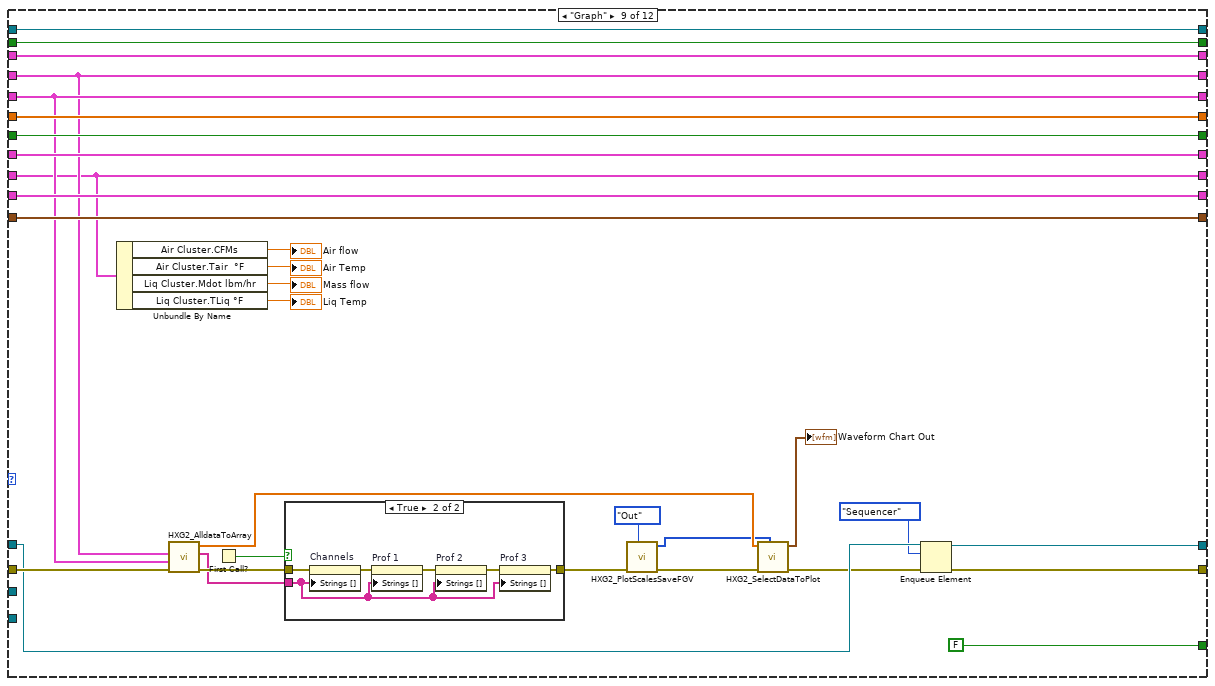
[diagram p13: hidden frame]
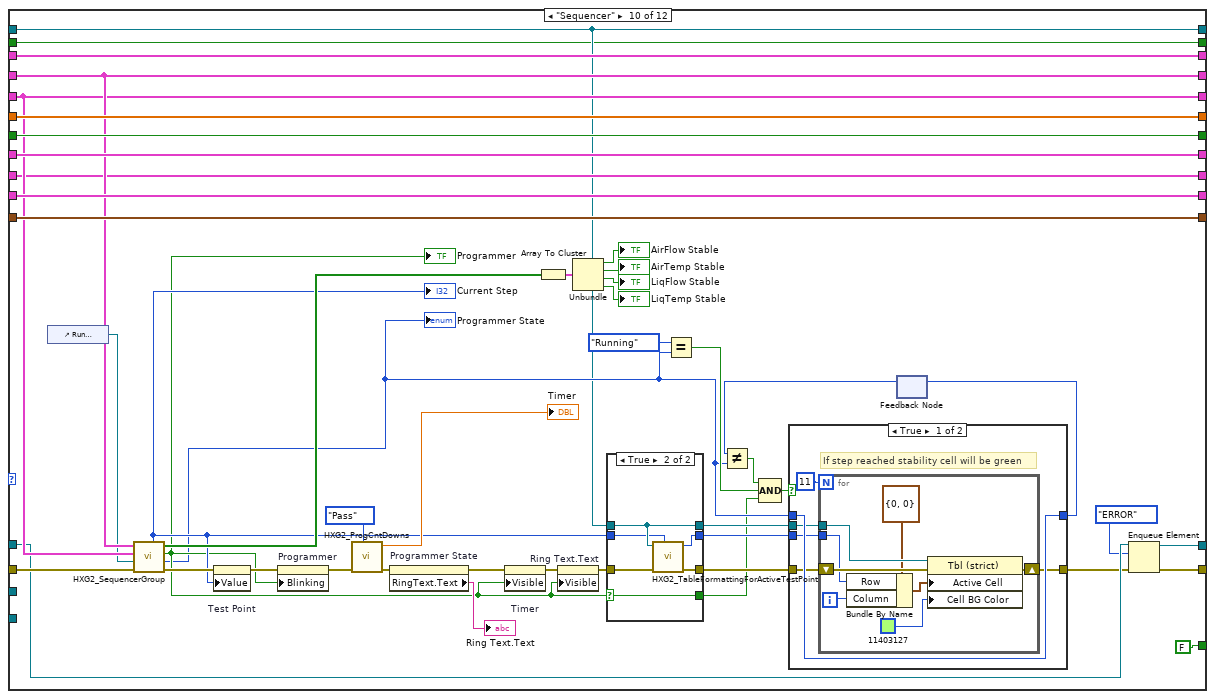
[diagram p15: hidden frame]
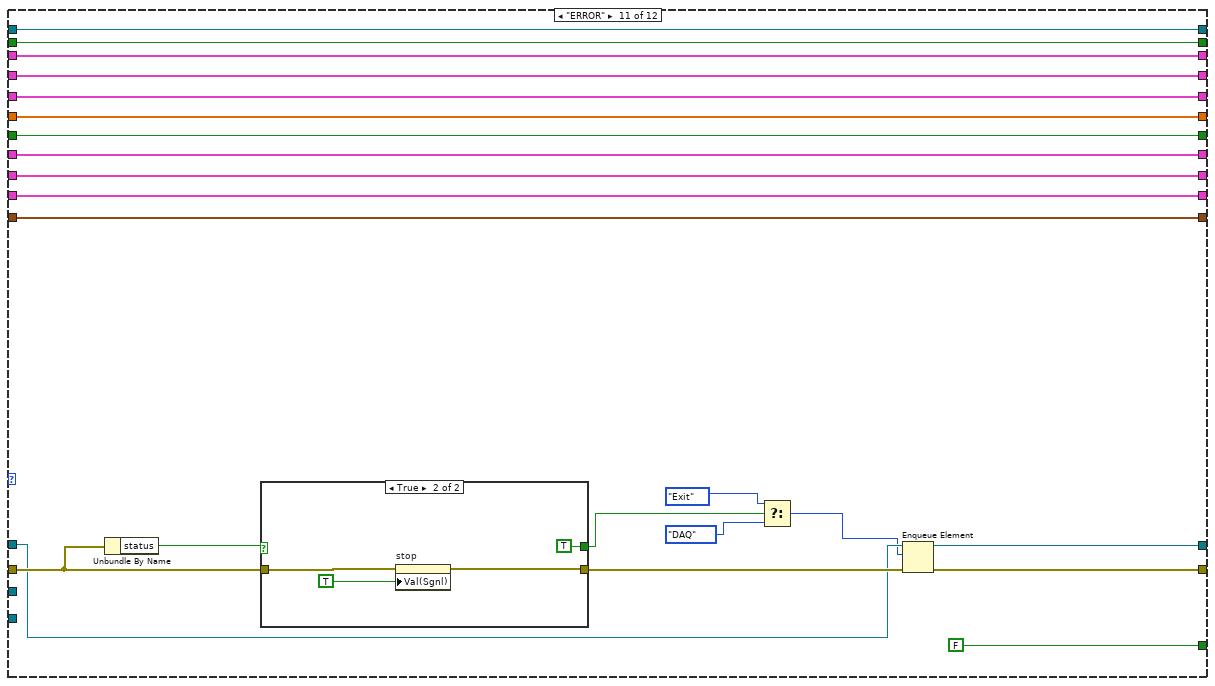
[diagram p18: hidden frame]
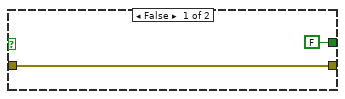
[diagram p19: hidden frame]
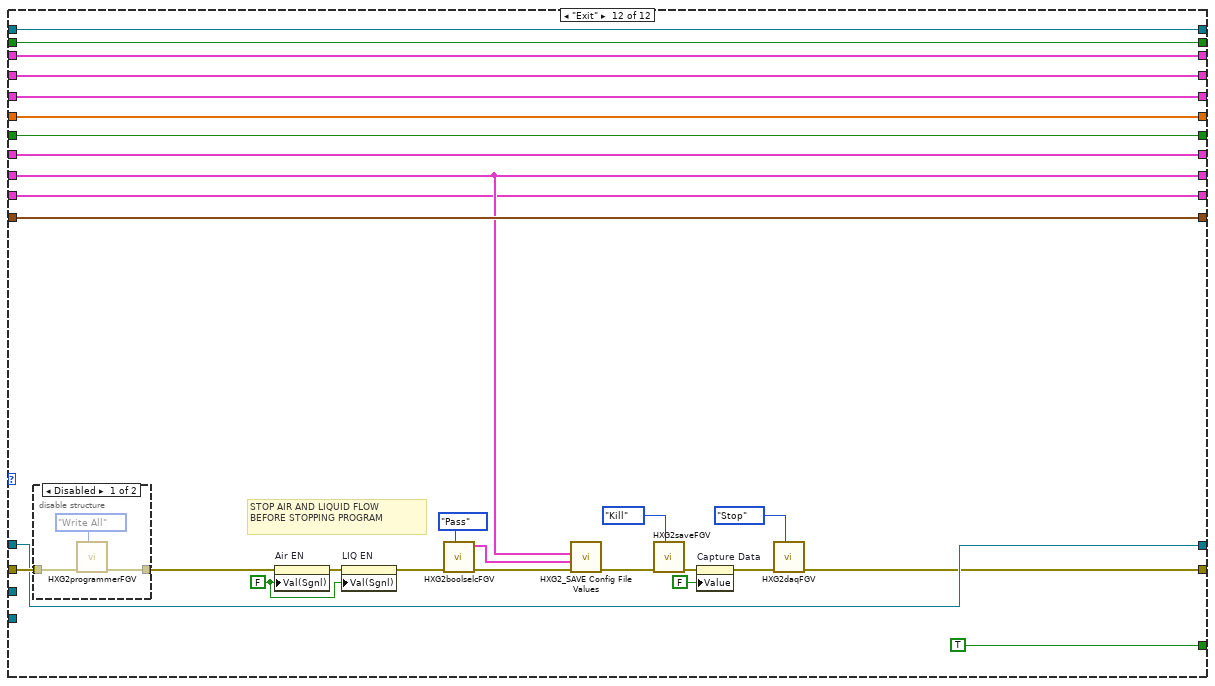
[diagram p20: hidden frame]
diagram:
  (unwired) errorcluster {"status"=FALSE, "code"=0, "source"=""} ("error out")
  w24 = HXG2_MainStateCtrl."Initialize" ("Main State Ctrl")
  w39 = T22 1 items=["no dialog", "OK message", "continue or stop message", "OK message + warnings", "continue/stop + warnings"] ("type of dialog (OK msg:1)")
  n1 = flat-sequence {
    tunnel: [w41] -> w19
    tunnel: "error in (no error)" -> [w49]
    frame #0 {
      w40 = FALSE ("stop")
      n2 = call "HXG2stopFGV.vi"("stopFGV"=HXG2stop."Write", "error in (no error)"=w49, "STOP"=w40) -> ("error out"=w47:errorcluster)  [unwired: 7 in, 1 out]
      n3 = local write "stop"(w40) -> ()
      n4 = property on="Air EN" class="Bool (strict)"(error in=w47, "Value"=w40) -> (error out=w46:errorcluster)  [unwired: 1 in, 1 out]
      n5 = property on="LIQ EN" class="Bool (strict)"(error in=w46, "Value"=w40) -> (error out=w45:errorcluster)  [unwired: 1 in, 1 out]
      n6 = property on="Run Programmer" class="Bool (strict)"(error in=w45, "Value"=w40) -> (error out=w44:errorcluster)  [unwired: 1 in, 1 out]
      n7 = property on="saving..." class="Bool (strict)"(error in=w44, "Value"=w40) -> (error out=w43:errorcluster)  [unwired: 1 in, 1 out]
      n8 = property on="Capture Data" class="Bool (strict)"(error in=w43, "Val(Sgnl)"=w40) -> (error out=w42:errorcluster)  [unwired: 1 in, 1 out]
      n9 = property on="Master RUN" class="Bool (strict)"(error in=w42, "Val(Sgnl)"=w40) -> (error out=w41:errorcluster)  [unwired: 1 in, 1 out]
    }
  }
  n10 = Obtain Queue(name (unnamed)="Main", element data type=w24, error in (no error)=w19) -> (queue out=w29:refnum<queue>, error out=w30:errorcluster)  [unwired: 2 in, 1 out]
  n11 = Obtain Queue(name (unnamed)="DAQ", element data type=HXG2_DAQLOOPctrl."Stop" ("DAQ Control"), error in (no error)=w19) -> (queue out=w34:refnum<queue>, error out=w33:errorcluster)  [unwired: 2 in, 1 out]
  n12 = Create User Event(user event datatype=errorcluster {"status"=FALSE, "code"=0, "source"=""} ("error out"), error in=w19) -> (user event=w12:refnum<user-event>, error out=w18:errorcluster)
  n13 = Enqueue Element(queue=w29, element=w24, error in (no error)=w30) -> (queue out=w26:refnum<queue>, error out=w27:errorcluster)  [unwired: 1 in, 1 out]
  n14 = Enqueue Element(queue=w34, element=HXG2_DAQLOOPctrl."Initialize" ("DAQ Control"), error in (no error)=w33) -> (queue out=w22:refnum<queue>, error out=w32:errorcluster)  [unwired: 1 in, 1 out]
  n15 = register-events(error in=w18, w12) -> (reference out=w16:refnum<event-registration>, error out=w17:errorcluster)  [unwired: 1 in]
  n16 = while {
    shift-right: [w54] -> w8
    shift-left: w17 -> [w58]
    tunnel: [w56] -> _
    tunnel: [w55] -> _
    tunnel: w16 -> [w51]
    tunnel: [w50] -> w13
    i -> [w57]
    stop <- w52 stop-if-true
    n17 = event shown="[21] \"Save Profile\", \"Load Profile\", \"Run Programmer\", \"Done Stop\", \"Repeat Execution:\", \"Table\": Value Change" {
      selector: w51 -> [_ _ _ _ _ _ _ _ _ _ _ _ _ _ _ _ _ _ _ _ _ _ _]
      dyn-events: [_ _ _ _ _ _ _ _ _ _ _ _ _ _ _ _ _ _ _ _ _ _ _] -> w50
      timeout: _ -> [_ _ _ _ _ _ _ _ _ _ _ _ _ _ _ _ _ _ _ _ _ _ _]
      tunnel: [FALSE FALSE ("stop") _ _ _ FALSE ("stop") "stop" TRUE ("stop") FALSE ("stop") _ FALSE _ _ FALSE ("stop") FALSE ("stop") _ _ _ FALSE ("stop") FALSE ("stop") FALSE ("stop") FALSE ("stop") _] -> w52
      tunnel: w58 -> [w59 w75 w155 w180 w181 w210 w219 w234 w244 w288 w296 w349 w352 w361 w381 w384 w393 w405 w414 w438 w498 w526 w567]
      tunnel: [w59 w77 w142 w179 w189 w204 w221 w234 w249 w287 w302 w345 w351 w354 w380 w386 w392 w404 w406 w435 w497 w533 w570] -> w53
      tunnel: [_ _ _ _ _ _ w227 _ _ _ _ _ _ _ _ _ _ _ _ _ _ _ _] -> w56
      tunnel: [_ _ _ _ _ _ w220 _ _ _ _ _ _ _ _ _ _ _ _ _ _ _ _] -> w55
      event Timeout {
        n18 = event-data() -> ()  [unwired: 1 in, 2 out]
      }
      event Value Change {
        w61 = T14 {"AF"=FALSE, "AC"=FALSE, "AH"=FALSE, "LF"=FALSE, "LC"=FALSE, "LH"=FALSE}  # Reset PIDs
        # "-SWITCH FROM PID TO MANUAL OPERATION WHEN AIR AND LIQ ARE\nSTOPPED\n- Start timers to detect drive malfunction when AIR and LIQ are ENABLED"
        n19 = event-data() -> ()  [unwired: 1 in, 2 out]
        n20 = call "HXG2enableFGV.vi"("ENABLE Ctrl"=HXG2enable."Pass", "error in (no error)"=w75) -> ("error out"=w74:errorcluster, "Air-Liq Out"=w72:bool[])  [unwired: 7 in, 1 out]
        n21 = control-ref of="AF PID"() -> (w83:refnum<vi>)
        n22 = control-ref of="AT PID"() -> (w82:refnum<vi>)
        n23 = control-ref of="LF PID"() -> (w80:refnum<vi>)
        n24 = control-ref of="LT PID"() -> (w79:refnum<vi>)
        n25 = Index Array(array=w72, index #1=0 ("index"), index #2=1 ("index")) -> (element #1=w68:bool, element #2=w69:bool)
        n26 = Compound Arithmetic op=AND("Air EN", invert w68) -> (w66:T9)
        n27 = Compound Arithmetic op=AND("LIQ EN", invert w69) -> (w67:T10)
        n28 = Build Array(w83, w82) -> (w81:refnum<vi>[])
        n29 = Build Array(w80, w79) -> (w78:refnum<vi>[])
        n30 = call "HXG2enableFGV.vi"("ENABLE Ctrl"=HXG2enable."Write" ("ENABLE"), "error in (no error)"=w74, "LIQ EN"="LIQ EN", "Air EN"="Air EN") -> ("error out"=w84:errorcluster)  [unwired: 5 in, 2 out]
        n31 = case shown="True" "LIQ EN" {
          tunnel: w84 -> [w123 w134]
          tunnel: [w121 w135] -> w63
          tunnel: w78 -> [_ w132]
          tunnel: w67 -> [w120 _]
          tunnel: w61 -> [w119 _]
          frame True {
            n32 = call "HXG2_Timing Module Pump.vi"("Timer Command"=HXG2_BlowerPumpl."Start", "error in (no error)"=w123) -> ("error out"=w122:errorcluster)  [unwired: 7 in, 2 out]
            n33 = case shown="True" w120 {
              selector: w120 -> [_ w126]
              tunnel: w122 -> [w125 w130]
              tunnel: [w125 w129] -> w121
              tunnel: w119 -> [_ w128]
              frame False {
              }
              frame True {
                n34 = Bundle By Name(cluster=w128, "LF"=w126, "LC"=w126, "LH"=w126) -> (w127:T14)
                n35 = call "HXG2pidFGV_gainscheduling.vi"("error in (no error)"=w130, "Reset PIDs"=w127, "PIDfgvCtrl"=HXG2pid."Wrt PID Resets") -> ("error out"=w129:errorcluster)  [unwired: 8 in, 8 out]
              }
            }
          }
          frame False {
            n36 = for {
              shift-right: [w139] -> w133
              shift-left: w134 -> [w140]
              tunnel: w132 -> [w138] mode=indexing
              n37 = property class="Bool (strict)"(reference=w138, error in=w140, "Val(Sgnl)"=FALSE ("stop")) -> (error out=w139:errorcluster)  [unwired: 1 out]
            }
            n38 = call "HXG2_Timing Module Pump.vi"("Timer Command"=HXG2_BlowerPumpl."Stop", "error in (no error)"=w133) -> ("error out"=w135:errorcluster)  [unwired: 7 in, 2 out]
          }
        }
        n39 = case shown="True" "Air EN" {
          tunnel: w63 -> [w97 w112]
          tunnel: [w96 w113] -> w62
          tunnel: w81 -> [_ w110]
          tunnel: w66 -> [w94 _]
          tunnel: w61 -> [w93 _]
          frame True {
            n40 = call "HXG2_Timing Module Blower.vi"("Timer Command"=HXG2_BlowerPumpl."Start", "error in (no error)"=w97) -> ("error out"=w95:errorcluster)  [unwired: 7 in, 2 out]
            n41 = case shown="True" w94 {
              selector: w94 -> [_ w100]
              tunnel: [w99 w104] -> w96
              tunnel: w95 -> [w99 w108]
              tunnel: w93 -> [_ w101]
              frame False {
              }
              frame True {
                w106 = TRUE ("Blinking")
                n42 = Bundle By Name(cluster=w101, "AF"=w100, "AC"=w100, "AH"=w100) -> (w102:T14)
                n43 = call "HXG2pidFGV_gainscheduling.vi"("error in (no error)"=w108, "Reset PIDs"=w102, "PIDfgvCtrl"=HXG2pid."Wrt PID Resets") -> ("error out"=w103:errorcluster)  [unwired: 8 in, 8 out]
                n44 = property on="HX ID" class="Str"(error in=w103, "Blinking"=w106) -> (error out=w107:errorcluster, "Caption"=w105:refnum<vi>)  [unwired: 1 in, 1 out]
                n45 = property class="Txt"(reference=w105, error in=w107, "Visible"=w106) -> (error out=w104:errorcluster)  [unwired: 1 out]
              }
            }
          }
          frame False {
            n46 = for {
              shift-right: [w117] -> w111
              shift-left: w112 -> [w118]
              tunnel: w110 -> [w116] mode=indexing
              n47 = property class="Bool (strict)"(reference=w116, error in=w118, "Val(Sgnl)"=FALSE ("stop")) -> (error out=w117:errorcluster)  [unwired: 1 out]
            }
            n48 = call "HXG2_Timing Module Blower.vi"("Timer Command"=HXG2_BlowerPumpl."Stop", "error in (no error)"=w111) -> ("error out"=w113:errorcluster)  [unwired: 7 in, 2 out]
          }
        }
        n49 = Or(x="Air EN", y="LIQ EN") -> (x .or. y?=w76:T9)
        n50 = case shown="False" w76 {
          selector: w76 -> [_ w90]
          tunnel: w62 -> [w89 w92]
          tunnel: [w88 w91] -> w77
          frame True {
            n51 = property on="Master RUN" class="Bool (strict)"(error in=w89, "Value"=TRUE ("Master RUN")) -> (error out=w88:errorcluster)  [unwired: 1 in, 1 out]
          }
          frame False {
            n52 = property on="Master RUN" class="Bool (strict)"(error in=w92, "Value"=w90) -> (error out=w91:errorcluster)  [unwired: 1 in, 1 out]
          }
        }
      }
      event "Set Prof 1", "Set Prof 2", "Set Prof 3": Value Change {
        w149 = u16[] [1, 43, 44, 7, 12, 40, 41, 27, 26, 37] items=["none", "Liq In Avg", "Liq In 1", "Liq In 2", "Liq Out Avg", "Liq Out 1", "Liq Out 2", "Fltrd Mdot", "Liq Mdot", "Liq T° f/mtr", "Liq dP 0-25psi", "Liq Pin 0-100psi", "Air In Avg", "Air In 1", "Air In 2", "Air In 3", "Air In 4", "Air Out Avg", "Air Out 1", "Air Out 2", "Air Out 3", "Air Out 4", "Air Out 5", "Air Out 6", "Air Out 7", "Air Out 8", "CFM Nozzle", "CFM HX", "UUT 0-0.1inWC x100", "Chmb 0-5inWC x100", "Chmb 0-2.5inWC x100", "Liq Q (BTU/hr)", "Liq Q (W)", "Air Q (BTU/hr)", "Air Q (W)", "SH (°F)", "SH multiplier", "%Energy Bal", "Liq Re", "AF Ctl Out", "AC Ctl Out", "AH Ctl Out", "LF Ctl Out", "LC Ctl Out", "LH Ctl Out"] ("Plot Selection")
        # "GRAPH PROFILES"
        n53 = event-data() -> ()  [unwired: 1 in, 5 out]
        n54 = case shown="True" "Set Prof 1" {
          tunnel: w155 -> [w173 w174]
          tunnel: [w173 w176] -> w154
          frame False {
          }
          frame True {
            n55 = property on="Plot Selection" class="Arr (strict)"(error in=w174, "Value"="Prof 1") -> (error out=w176:errorcluster)  [unwired: 1 in, 1 out]
          }
        }
        n56 = control-ref of="Set Prof 1"() -> (w147:refnum<vi>)
        n57 = control-ref of="Set Prof 2"() -> (w146:refnum<vi>)
        n58 = control-ref of="Set Prof 3"() -> (w145:refnum<vi>)
        n59 = control-ref of="Default"() -> (w144:refnum<vi>)
        n60 = Build Array(w147, w146, w145, w144) -> (w141:refnum<vi>[])
        n61 = case shown="True" "Set Prof 2" {
          tunnel: w154 -> [w169 w170]
          tunnel: [w169 w172] -> w151
          frame False {
          }
          frame True {
            n62 = property on="Plot Selection" class="Arr (strict)"(error in=w170, "Value"="Prof 2") -> (error out=w172:errorcluster)  [unwired: 1 in, 1 out]
          }
        }
        n63 = case shown="True" "Set Prof 3" {
          tunnel: w151 -> [w165 w166]
          tunnel: [w165 w168] -> w150
          frame False {
          }
          frame True {
            n64 = property on="Plot Selection" class="Arr (strict)"(error in=w166, "Value"="Prof 3") -> (error out=w168:errorcluster)  [unwired: 1 in, 1 out]
          }
        }
        n65 = case shown="True" "Default" {
          tunnel: w150 -> [w161 w164]
          tunnel: [w161 w163] -> w143
          tunnel: w149 -> [_ w162]
          frame False {
          }
          frame True {
            n66 = property on="Plot Selection" class="Arr (strict)"(error in=w164, "Value"=w162) -> (error out=w163:errorcluster)  [unwired: 1 in, 1 out]
          }
        }
        n67 = for {
          shift-right: [w159] -> w142
          shift-left: w143 -> [w160]
          tunnel: w141 -> [w158] mode=indexing
          n68 = property class="Bool (strict)"(reference=w158, error in=w160, "Value"=FALSE ("Set Prof 2")) -> (error out=w159:errorcluster)  [unwired: 1 out]
        }
      }
      event "Plot Selection": Value Change {
        n69 = event-data() -> ()  [unwired: 1 in, 5 out]
        n70 = call "HXG2_PlotScalesSaveFGV.vi"(7:HXG2_GraphSelections."Plot Selection In", "error in (no error)"=w180, "Plot Selection In"="Plot Selection") -> ("error out"=w179:errorcluster)  [unwired: 4 in, 4 out]
      }
      event "TC 1", "TC 2", "TC 3", "TC 4", "TC 5", "TC 6", "TC 7", "TC 8": Value Change {
        n71 = event-data() -> ()  [unwired: 1 in, 5 out]
        n72 = Build Array("TC 1", "TC 2", "TC 3", "TC 4", "TC 5", "TC 6", "TC 7", "TC 8") -> (w182:string[])
        n73 = property on="Channels" class="Ring (strict)"(error in=w181) -> (error out=w187:errorcluster, "Strings []"=w188:string[])  [unwired: 1 in, 1 out]
        n74 = Build Array (concatenate)(w188, w182) -> (w186:string[])
        n75 = property on="Channels" class="Ring (strict)"(error in=w187, "Strings []"=w186) -> (error out=w185:errorcluster)  [unwired: 1 in, 1 out]
        n76 = property on="Prof 1" class="Ring (strict)"(error in=w185, "Strings []"=w186) -> (error out=w184:errorcluster)  [unwired: 1 in, 1 out]
        n77 = property on="Prof 2" class="Ring (strict)"(error in=w184, "Strings []"=w186) -> (error out=w183:errorcluster)  [unwired: 1 in, 1 out]
        n78 = property on="Prof 3" class="Ring (strict)"(error in=w183, "Strings []"=w186) -> (error out=w189:errorcluster)  [unwired: 1 in, 1 out]
      }
      event "Master RUN": Value Change {
        n79 = event-data() -> ()  [unwired: 1 in, 5 out]
        n80 = case shown="False" "Master RUN" {
          tunnel: w210 -> [w216 w218]
          tunnel: [w216 w218] -> w207
          tunnel: [FALSE ("stop") TRUE ("stop")] -> w198
          frame False {
          }
          frame True {
          }
        }
        n81 = control-ref of="LF PID"() -> (w203:refnum<vi>)
        n82 = control-ref of="LT PID"() -> (w202:refnum<vi>)
        n83 = control-ref of="AF PID"() -> (w201:refnum<vi>)
        n84 = control-ref of="AT PID"() -> (w200:refnum<vi>)
        n85 = property on="Air EN" class="Bool (strict)"(error in=w207, "Val(Sgnl)"=w198) -> (error out=w206:errorcluster)  [unwired: 1 in, 1 out]
        n86 = Build Array(w203, w202, w201, w200) -> (w199:refnum<vi>[])
        n87 = property on="LIQ EN" class="Bool (strict)"(error in=w206, "Val(Sgnl)"=w198) -> (error out=w205:errorcluster)  [unwired: 1 in, 1 out]
        n88 = for {
          shift-right: [w213] -> w204
          shift-left: w205 -> [w214]
          tunnel: w199 -> [w212] mode=indexing
          tunnel: w198 -> [w211]
          n89 = property class="Bool (strict)"(reference=w212, error in=w214, "Val(Sgnl)"=w211) -> (error out=w213:errorcluster)  [unwired: 1 out]
        }
      }
      event "stop": Value Change {
        w224 = HXG2_DAQLOOPctrl."Stop" ("DAQ Control")
        w229 = HXG2_MainStateCtrl."Exit" ("Main State Ctrl")
        n90 = event-data() -> ()  [unwired: 1 in, 5 out]
        n91 = Obtain Queue(name (unnamed)="Main", element data type=w229, error in (no error)=w219) -> (queue out=w231:refnum<queue>, error out=w228:errorcluster)  [unwired: 2 in, 1 out]
        n92 = Enqueue Element At Opposite End(queue=w231, element=w229, error in (no error)=w228) -> (queue out=w227:refnum<queue>, error out=w223:errorcluster)  [unwired: 1 in, 1 out]
        n93 = Obtain Queue(name (unnamed)="DAQ", element data type=w224, error in (no error)=w223) -> (queue out=w226:refnum<queue>, error out=w222:errorcluster)  [unwired: 2 in, 1 out]
        n94 = Enqueue Element(queue=w226, element=w224, error in (no error)=w222) -> (queue out=w220:refnum<queue>, error out=w221:errorcluster)  [unwired: 1 in, 1 out]
      }
      event User Event {
        # "STOP IF THERE IS AN ERROR"
        n95 = event-data() -> ()  [unwired: 1 in, 6 out]
      }
      event "LiqIn 1 °F", "LiqIn 2 °F", "LiqOut 1 °F", "LiqOut 2 °F", "AirIn 1 °F", "AirIn 2 °F", "AirIn 3 °F", "AirIn 4 °F", "AirOut 1 °F", "AirOut 2 °F", "AirOut 3 °F", "AirOut 4 °F", "AirOut 5 °F", "AirOut 6 °F", "AirOut 7 °F", "AirOut 8 °F", "0.75\"", "1\"", "1.25\"", "1.5\"", "Tube ID (in)", "Select Tube OD", "Sensor", "Fan TR", "Fan TL", "Fan BL", "Fan BR": Value Change {
        n96 = event-data() -> ()  [unwired: 1 in, 5 out]
        n97 = case shown="4" "Select Tube OD" {
          tunnel: w244 -> [w273 w275 w278 w281 w286]
          tunnel: [w273 w275 w278 w281 w285] -> w242
          tunnel: [0.315 ("Tube ID (in)") 0.272 ("Tube ID (in)") 0.21 ("Tube ID (in)") 0.188 ("Tube ID (in)") "Tube ID (in)"] -> w243
          tunnel: [FALSE ("Visible") FALSE ("Visible") FALSE ("Visible") FALSE ("Visible") w283] -> w240
          frame 0, Default {
            # "3/8"
          }
          frame 1 {
            # "5/16"
          }
          frame 2 {
            # "1/4"
          }
          frame 3 {
            # "3/16"
          }
          frame 4 {
            w283 = TRUE ("Visible")
            n98 = property on="Tube ID (in)" class="DigNum (strict)"(error in=w286, "Visible"=w283) -> (error out=w285:errorcluster)  [unwired: 1 in, 1 out]
          }
        }
        n99 = property on="Tube ID (in)" class="DigNum (strict)"(error in=w242, "Visible"=w240) -> (error out=w241:errorcluster)  [unwired: 1 in, 1 out]
        n100 = Bundle By Name(cluster=T29 {"Bool"={"Use GlyIn 1"=FALSE, "Use GlyIn 2"=FALSE, "Use GlyOut 1"=FALSE, "Use GlyOut 2"=FALSE, "Use AirIn 1"=FALSE, "Use AirIn 2"=FALSE, "Use AirIn 3"=FALSE, "Use AirIn 4"=FALSE, "Use AirOut 1"=FALSE, "Use AirOut 2"=FALSE, "Use AirOut 3"=FALSE, "Use AirOut 4"=FALSE, "Use AirOut 5"=FALSE, "Use AirOut 6"=FALSE, "Use AirOut 7"=FALSE, "Use AirOut 8"=FALSE, "0.75in Nozzle"=FALSE, "1.00in Nozzle"=FALSE, "1.25in Nozzle"=FALSE, "1.5in Nozzle"=FALSE, "On 2.5inWC/Off 5inWC"=FALSE, "Fan TR"=FALSE, "Fan TL"=FALSE, "Fan BR"=FALSE, "Fan BL"=FALSE}, "Other"={"Tube ID"=0.0}} ("Bools"), "Bool.Fan TR"="Fan TR", "Bool.Fan TL"="Fan TL", "Bool.Fan BR"="Fan BR", "Bool.Fan BL"="Fan BL", "Bool.Use GlyIn 1"="LiqIn 1 °F", "Bool.Use GlyIn 2"="LiqIn 2 °F", "Bool.Use GlyOut 1"="LiqOut 1 °F", "Bool.Use GlyOut 2"="LiqOut 2 °F", "Bool.Use AirIn 1"="AirIn 1 °F", "Bool.Use AirIn 2"="AirIn 2 °F", "Bool.Use AirIn 3"="AirIn 3 °F", "Bool.Use AirIn 4"="AirIn 4 °F", "Bool.Use AirOut 1"="AirOut 1 °F", "Bool.Use AirOut 2"="AirOut 2 °F", "Bool.Use AirOut 3"="AirOut 3 °F", "Bool.Use AirOut 4"="AirOut 4 °F", "Bool.Use AirOut 5"="AirOut 5 °F", "Bool.Use AirOut 6"="AirOut 6 °F", "Bool.Use AirOut 7"="AirOut 7 °F", "Bool.Use AirOut 8"="AirOut 8 °F", "Bool.0.75in Nozzle"="0.75\"", "Bool.1.00in Nozzle"="1\"", "Bool.1.25in Nozzle"="1.25\"", "Bool.1.5in Nozzle"="1.5\"", "Bool.On 2.5inWC/Off 5inWC"="Sensor", "Other.Tube ID"=w243) -> (w247:T29)
        n101 = call "HXG2boolselcFGV.vi"("BoolselecFGV"=HXG2boolselec."Write", "error in (no error)"=w241, "Boolean Selections"=w247) -> ("error out"=w249:errorcluster)  [unwired: 7 in, 1 out]
      }
      event "Liq Tin (°F)", "Target Re", "HX ID (in)": Value Change {
        n102 = event-data() -> ()  [unwired: 1 in, 5 out]
        n103 = call "HXG2_Re-Calc.vi"("error in (no error)"=w288, "Tube ID (in)"="HX ID (in)", "Target Re"="Target Re", "Liq Tin (°F)"="Liq Tin (°F)") -> ("error out"=w287:errorcluster, "Cp (BTU/lbm°F)"=→"Cp (BTU/lbm°F)":dbl, "Density (lbm/ft³)"=→"Density (lbm/ft³)":dbl, "mdot (lbm/hr)"=→"mdot (lbm/hr)":dbl, "mu (lbm/ft*s)"=→"mu (lbm/ft*s)":dbl)  [unwired: 3 in]
      }
      event "Capture Data": Value Change {
        n104 = event-data() -> ("OldVal"=w299:bool)  [unwired: 1 in, 4 out]
        n105 = call "HXG2saveFGV.vi"("saveFGV"=HXG2save."Write", "error in (no error)"=w296, "Capture Data"="Capture Data") -> ("error out"=w298:errorcluster, "Saving?"=w297:bool)  [unwired: 4 in, 3 out]
        n106 = Compound Arithmetic op=AND(invert w299, w297) -> (w303:bool)
        n107 = case shown="True" w303 {
          tunnel: w298 -> [w311 w333]
          tunnel: [w310 w336] -> w302
          tunnel: w297 -> [w309 _]
          tunnel: "Duration Ctrl" -> [w306 w341]
          tunnel: w299 -> [w308 _]
          frame False {
            n108 = Compound Arithmetic op=AND(w308, invert w309) -> (w307:bool)
            n109 = case shown="True" w307 {
              tunnel: w311 -> [w315 w325]
              tunnel: [w314 w327] -> w310
              tunnel: w306 -> [w312 _]
              frame False {
                n110 = call "HXG2saveTimer.vi"("SaveTimerFGV"=HXG2saveTimer."EvntStrtDurtn", "error in (no error)"=w315, "Duration(min)"=w312) -> ("error out"=w314:errorcluster)  [unwired: 4 in, 4 out]
              }
              frame True {
                n111 = call "HXG2saveFGV.vi"("saveFGV"=HXG2save."Pass", "error in (no error)"=w325) -> ("error out"=w320:errorcluster, "tdms file out"=w319:refnum<k34>)  [unwired: 5 in, 3 out]
                n112 = call "HXG2_CoilDataFGV.vi"("FGVctrl"=enum16{"Write", "Pass"}."Pass", "error in (no error)"=w320) -> ("error out"=w323:errorcluster, "Header"=w324:string[], "Data Out"=w318:string[])  [unwired: 7 in]
                n113 = TDMS Set Properties(5:w318, 7:w324, 8:w323, 10:"General Data" ("group name in (Untitled)"), 11:w319) -> (0:w316:errorcluster, 3:w317:refnum<k34>)  [unwired: 1 in, 2 out]
                n114 = call "HXG2saveFGV.vi"("saveFGV"=HXG2save."Kill", "error in (no error)"=w316, "tdms ref In"=w317) -> ("error out"=w329:errorcluster)  [unwired: 4 in, 4 out]
                n115 = call "HXG2saveTimer.vi"("SaveTimerFGV"=HXG2saveTimer."Stop", "error in (no error)"=w329) -> ("error out"=w327:errorcluster)  [unwired: 5 in, 4 out]
              }
            }
          }
          frame True {
            n116 = property on="HX ID" class="Str"(error in=w333) -> (error out=w332:errorcluster, "Value"=w331:string)  [unwired: 1 in, 1 out]
            n117 = call "HXG2saveFGV.vi"("saveFGV"=HXG2save."Initialize", "error in (no error)"=w332, "HX Description"=w331) -> ("error out"=w343:errorcluster)  [unwired: 4 in, 4 out]
            n118 = call "HXG2saveTimer.vi"("SaveTimerFGV"=HXG2saveTimer."EvntStrtDurtn", "error in (no error)"=w343, "Duration(min)"=w341) -> ("error out"=w340:errorcluster)  [unwired: 4 in, 4 out]
            n119 = property on="Interval Ctrl" class="DigNum (strict)"(error in=w340) -> (error out=w339:errorcluster, "Value"=w337:dbl)  [unwired: 1 in, 1 out]
            n120 = call "HXG2saveTimer.vi"("SaveTimerFGV"=HXG2saveTimer."EvntStrtInterv", "error in (no error)"=w339, "Interval(s)"=w337) -> ("error out"=w334:errorcluster)  [unwired: 4 in, 4 out]
            n121 = property on="File Name" class="Str"(error in=w334, "Visible"=TRUE) -> (error out=w336:errorcluster)  [unwired: 1 in, 1 out]
          }
        }
      }
      event "HX ID": Value Change; "HX ID": Mouse Down {
        w347 = FALSE ("Blinking")
        # "BLINKING OF THE HX ID STRING CONTROL should start as soon as AIR or LIQ are enabled.\nIf the user types a new name of clicks on the control, we will assume that the name is accepted\nthis name is used in the save file name."
        n122 = event-data() -> ()  [unwired: 1 in, 3 out]
        n123 = property on="HX ID" class="Str"(error in=w349, "Blinking"=w347) -> (error out=w346:errorcluster, "Caption"=w348:refnum<vi>)  [unwired: 1 in, 1 out]
        n124 = property class="Txt"(reference=w348, error in=w346, "Visible"=w347) -> (error out=w345:errorcluster)  [unwired: 1 out]
      }
      event "Select Path": Value Change {
        n125 = event-data() -> ()  [unwired: 1 in, 5 out]
        n126 = call <vilib>:"TDMS - File Viewer.vi"("error in (no error)"=w352, "file path"="Select Path") -> ("error out"=w351:errorcluster)  [unwired: 5 out]
      }
      event "Interval Ctrl", "+10", "-10": Value Change {
        n127 = event-data() -> ()  [unwired: 1 in, 5 out]
        n128 = call "HXG2saveTimer.vi"("SaveTimerFGV"=HXG2saveTimer."EvntStrtInterv", "error in (no error)"=w361, "Interval(s)"="Interval Ctrl") -> ("error out"=w355:errorcluster)  [unwired: 4 in, 4 out]
        n129 = Or(x="+10", y="-10") -> (x .or. y?=w356:bool)
        n130 = case shown="True" w356 {
          tunnel: [w362 w371] -> w354
          tunnel: w355 -> [w362 w375]
          tunnel: "+10" -> [_ w366]
          frame False {
          }
          frame True {
            n131 = Select(t=10.0, s=w366, f=-10.0 ("t")) -> (s? t:f=w363:dbl)
            n132 = Select(t=HXG2saveTimer."Add10Durtn" ("SaveTimerFGV"), s=w366, f=HXG2saveTimer."Take10Durtn" ("SaveTimerFGV")) -> (s? t:f=w372:T31)
            n133 = call "HXG2saveTimer.vi"("SaveTimerFGV"=w372, "error in (no error)"=w375) -> ("error out"=w370:errorcluster)  [unwired: 5 in, 4 out]
            n134 = property on="Duration Ctrl" class="DigNum (strict)"(error in=w370) -> (error out=w368:errorcluster, "Value"=w367:dbl)  [unwired: 1 in, 1 out]
            n135 = Add(x=w367, y=w363) -> (x+y=w369:dbl)
            n136 = property on="Duration Ctrl" class="DigNum (strict)"(error in=w368, "Value"=w369) -> (error out=w371:errorcluster)  [unwired: 1 in, 1 out]
          }
        }
      }
      event Value Change {
        n137 = event-data() -> ()  [unwired: 1 in, 5 out]
        n138 = call "HXG2air-glyClusterFGV.vi"("AirGlyCtrl"=HXG2airglyCluster."Write", "error in (no error)"=w381, "Gly Cluster"="Liq Cluster", "Air Cluster"="Air Cluster") -> ("error out"=w380:errorcluster)  [unwired: 6 in, 1 out]
      }
      event Value Change {
        n139 = event-data() -> ()  [unwired: 1 in, 5 out]
        n140 = call "HXG2pidFGV_gainscheduling.vi"("AirCool Cascade"="AirCool Cascade", "LiqHeat Cascade"="LiqHeat Cascade", "PID gains in"="PID Setup Array", "error in (no error)"=w384, "PIDfgvCtrl"=HXG2pid."Write PID Gains") -> ("error out"=w389:errorcluster)  [unwired: 6 in, 8 out]
        n141 = call "HXG2pidFGV_gainscheduling.vi"("error in (no error)"=w389, "PIDfgvCtrl"=HXG2pid."Pass") -> ("PID Gains Out"=w385:T12, "error out"=w387:errorcluster)  [unwired: 9 in, 7 out]
        n142 = call "HXG2_SAVE-PID_gains_gainscheduling.vi"("error in"=w387, "PID Setup Array"=w385) -> ("error out"=w386:errorcluster)  [unwired: 9 in]
      }
      event "SchedSelect", "PID Select": Value Change {
        n143 = event-data() -> ()  [unwired: 1 in, 5 out]
        n144 = Build Array("PID Select") -> (w400:T39)
        n145 = To Unsigned Long Integer(number=w400) -> (unsigned 32bit integer=w399:u32[])
        n146 = property on="PID Setup Array" class="Arr (strict)"(error in=w393, "Index Values"=w399) -> (error out=w398:errorcluster)  [unwired: 1 in, 1 out]
        n147 = Build Array("SchedSelect") -> (w396:T40)
        n148 = To Unsigned Long Integer(number=w396) -> (unsigned 32bit integer=w394:u32[])
        n149 = property on="GainsArray" class="Arr (strict)"(error in=w398, "Index Values"=w394) -> (error out=w395:errorcluster)  [unwired: 1 in, 1 out]
        n150 = property on="UL-LL Array" class="Arr (strict)"(error in=w395, "Index Values"=w394) -> (error out=w392:errorcluster)  [unwired: 1 in, 1 out]
      }
      event Value Change {
        n151 = event-data() -> ()  [unwired: 1 in, 5 out]
        n152 = call "HXG2pidFGV_gainscheduling.vi"("error in (no error)"=w405, "Reset PIDs"="Reset PIDs", "PIDfgvCtrl"=HXG2pid."Wrt PID Resets") -> ("error out"=w404:errorcluster)  [unwired: 8 in, 8 out]
      }
      event "Max 1", "Min 1", "Max 2", "Min 2", "Max 3", "Min 3", "x-axis length (min)", "Apply Scales", "Plot Axis": Value Change {
        w410 = TRUE ("Apply Scales")
        n153 = event-data() -> ()  [unwired: 1 in, 5 out]
        n154 = Build Array("x-axis length (min)", "Max 1", "Min 1", "Max 2", "Min 2", "Max 3", "Min 3") -> (w411:dbl[])
        n155 = call "HXG2_PlotScalesSaveFGV.vi"(7:HXG2_GraphSelections."Graph Scales In", "error in (no error)"=w414, "Apply Scales"=w410, "Scales In"=w411) -> ("error out"=w413:errorcluster)  [unwired: 3 in, 4 out]
        n156 = control-ref of="Waveform Chart Out"() -> (w415:refnum<vi>)
        n157 = call "HXG2_Grapher-Scales.vi"("Graph Scales In"=w411, "Update Chart"=w410, "Scale Ctrl"="Plot Axis", "error in (no error)"=w413, "Waveform Chart Ref in"=w415) -> ("error out"=w409:errorcluster)  [unwired: 10 in]
        n158 = call "HXG2_PlotScalesSaveFGV.vi"("Plot Axis In"="Plot Axis", 7:HXG2_GraphSelections."Plot Axis In", "error in (no error)"=w409) -> ("error out"=w406:errorcluster)  [unwired: 4 in, 4 out]
      }
      event "AF PID", "AT PID", "LF PID", "LT PID": Value Change {
        n159 = event-data() -> ("CtlRef"=w432:refnum<vi>, "OldVal"=w425:bool, "NewVal"=w434:bool)  [unwired: 1 in, 2 out]
        n160 = Bundle By Name(cluster=T33 {"AF PID"=FALSE, "AT PID"=FALSE, "LF PID"=FALSE, "LT PID"=FALSE} ("PIDon-off In"), "AF PID"="AF PID", "AT PID"="AT PID", "LF PID"="LF PID", "LT PID"="LT PID") -> (w437:T33)
        n161 = call "HXG2pidFGV_gainscheduling.vi"("PIDon-off In"=w437, "error in (no error)"=w438, "PIDfgvCtrl"=HXG2pid."Write PID On-Off") -> ("error out"=w431:errorcluster)  [unwired: 8 in, 8 out]
        n162 = call "HXG2pidFGV_gainscheduling.vi"("error in (no error)"=w431, "PIDfgvCtrl"=HXG2pid."Pass") -> ("PID Ctrls Out"=w428:T41, "PID Refs Out"=w424:T42, "error out"=w430:errorcluster)  [unwired: 9 in, 6 out]
        n163 = Compound Arithmetic op=AND(w425, invert w434) -> (w433:bool)
        n164 = case shown="True" w433 {
          tunnel: w430 -> [w443 w450]
          tunnel: [w443 w446] -> w435
          tunnel: w432 -> [_ w449]
          tunnel: w428 -> [_ w445]
          tunnel: w424 -> [_ w444]
          frame False {
          }
          frame True {
            # "STOP PID"
            n165 = property class="Bool (strict)"(reference=w449, error in=w450) -> (error out=w447:errorcluster, "BoolText.Text"=w448:string)  [unwired: 1 out]
            n166 = case shown="\"AF PID\"" w448 {
              tunnel: w447 -> [w451 w462 w472 w482 w493]
              tunnel: [w451 w458 w465 w475 w483] -> w446
              tunnel: w445 -> [_ w461 _ _ w492]
              tunnel: w444 -> [_ w457 w463 w474 w485]
              frame "False", Default {
              }
              frame "AF PID" {
                n167 = Unbundle By Name(w461) -> ("af ctrl effort"=w460:dbl)
                n168 = Unbundle By Name(w457) -> ("Reset Ctrls"=w456:refnum<vi>[])
                n169 = property on="Air FLOW %" class="DigNum (strict)"(error in=w462, "Val(Sgnl)"=w460) -> (error out=w459:errorcluster)  [unwired: 1 in, 1 out]
                n170 = Index Array(array=w456, index=0) -> (element=w454:refnum<vi>)
                n171 = To Variant(anything=TRUE ("Value (Signaling)")) -> (Variant=w452:variant)
                n172 = property class="Ctl"(reference=w454, error in=w459, "Val(Sgnl)"=w452) -> (error out=w458:errorcluster)  [unwired: 1 out]
              }
              frame "AT PID" {
                n173 = Unbundle By Name(w463) -> ("Reset Ctrls"=w464:refnum<vi>[])
                n174 = property on="Air TEMP %" class="DigNum (strict)"(error in=w472, "Val(Sgnl)"=50.0 ("Value (Signaling)")) -> (error out=w466:errorcluster)  [unwired: 1 in, 1 out]
                n175 = Index Array(array=w464, index=1) -> (element=w469:refnum<vi>)
                n176 = To Variant(anything=TRUE ("Value (Signaling)")) -> (Variant=w467:variant)
                n177 = property class="Ctl"(reference=w469, error in=w466, "Val(Sgnl)"=w467) -> (error out=w465:errorcluster)  [unwired: 1 out]
              }
              frame "LT PID" {
                n178 = Unbundle By Name(w474) -> ("Reset Ctrls"=w473:refnum<vi>[])
                n179 = property on="Liq TEMP %" class="DigNum (strict)"(error in=w482, "Val(Sgnl)"=50.0 ("Value (Signaling)")) -> (error out=w476:errorcluster)  [unwired: 1 in, 1 out]
                n180 = Index Array(array=w473, index=2) -> (element=w479:refnum<vi>)
                n181 = To Variant(anything=TRUE ("Value (Signaling)")) -> (Variant=w477:variant)
                n182 = property class="Ctl"(reference=w479, error in=w476, "Val(Sgnl)"=w477) -> (error out=w475:errorcluster)  [unwired: 1 out]
              }
              frame "LF PID" {
                n183 = Unbundle By Name(w485) -> ("Reset Ctrls"=w484:refnum<vi>[])
                n184 = Unbundle By Name(w492) -> ("lf ctrl effort"=w491:dbl)
                n185 = property on="Liq FLOW %" class="DigNum (strict)"(error in=w493, "Val(Sgnl)"=w491) -> (error out=w486:errorcluster)  [unwired: 1 in, 1 out]
                n186 = Index Array(array=w484, index=3) -> (element=w489:refnum<vi>)
                n187 = To Variant(anything=TRUE ("Value (Signaling)")) -> (Variant=w487:variant)
                n188 = property class="Ctl"(reference=w489, error in=w486, "Val(Sgnl)"=w487) -> (error out=w483:errorcluster)  [unwired: 1 out]
              }
            }
          }
        }
      }
      event "Reset Alarm UI": Value Change {
        # "This hidden button clears alarms on the HXG2 _ALARM Parser VI"
        n189 = event-data() -> ()  [unwired: 1 in, 5 out]
        n190 = case shown="True" "Reset Alarm UI" {
          tunnel: [w499 w503] -> w497
          tunnel: w498 -> [w499 w508]
          frame False {
          }
          frame True {
            w509 = FALSE ("Value (Signaling)")
            n191 = control-ref of="Alarm Set Button"() -> (w507:refnum<vi>)
            n192 = property class="Bool (strict)"(reference=w507, error in=w508, "Val(Sgnl)"=w509) -> (error out=w510:errorcluster)  [unwired: 1 out]
            n193 = control-ref of="Reset Alarm UI"() -> (w506:refnum<vi>)
            n194 = property class="Bool (strict)"(reference=w506, error in=w510, "Val(Sgnl)"=w509) -> (error out=w504:errorcluster)  [unwired: 1 out]
            n195 = Bundle By Name(cluster=T34 {"All Digital IN"={"LiqNotlow"=FALSE, "LiqHtrNotOverTemp"=FALSE, "AirHtrNotOverTemp"=FALSE, "BlowerVFD-On"=FALSE, "PumpVFD-On"=FALSE, "CompNotOverloaded"=FALSE, "CompNotOverPdisch"=FALSE, "EMOcleared"=FALSE, "EMOreset"=FALSE, "Master Power Switch"=FALSE, "HX Flood"=FALSE}} ("Digital In"), "All Digital IN.EMOreset"=TRUE ("All Digital IN.EMO Reset")) -> (w501:T34)
            n196 = call "HXG2DataTransFGV.vi"("DataTransCtrl"=HXG2DataTrans."Write", "error in (no error)"=w504, "Digital In"=w501) -> ("error out"=w503:errorcluster)  [unwired: 7 in, 1 out]
          }
        }
        "Clear Alarms" <- TRUE ("Clear Alarms")
      }
      event "Save Profile", "Load Profile", "Run Programmer", "Done Stop", "Repeat Execution:", "Table": Value Change {
        # "Stop Air & Liq\nwhen profile ends"
        # "Start saving and disable button \nif programmer starts"
        # "Update profile if table control is\nchanged"
        # "Stop saving if programmer stops"
        n197 = event-data() -> ()  [unwired: 1 in, 1 out]
        n198 = call "HXG2programmerFGV.vi"("Programmer Ctrl"=HXG2programmer."Pass All", "error in (no error)"=w526) -> ("error out"=w525:errorcluster, "User Selections Out"=w523:T37)  [unwired: 5 in, 3 out]
        n199 = Unbundle By Name(w523) -> ("Run Prog"=w530:bool)
        n200 = call "HXG2_ProgammerParseData.vi"("Parse Ctrl"=enum16{"Write", "Pass"}."Write", "error in (no error)"=w525, "Table Data In"="Table") -> ("error out"=w521:errorcluster)  [unwired: 7 in, 1 out]
        n201 = Compound Arithmetic op=AND("Run Programmer", invert w530) -> (w519:bool)
        n202 = Compound Arithmetic op=AND(invert "Run Programmer", w530) -> (w513:bool)
        n203 = case shown="True" w519 {
          tunnel: w521 -> [w544 w549]
          tunnel: [w544 w546] -> w520
          frame False {
          }
          frame True {
            n204 = property on="Capture Data" class="Bool (strict)"(error in=w549, "Val(Sgnl)"=TRUE ("Value (Signaling)")) -> (error out=w547:errorcluster)  [unwired: 1 in, 1 out]
            n205 = property on="Capture Data" class="Bool (strict)"(error in=w547, "DisabledEnum"=T38."Disabled and Grayed Out" ("Disabled")) -> (error out=w546:errorcluster)  [unwired: 1 in, 1 out]
          }
        }
        n206 = case shown="True" w513 {
          tunnel: w520 -> [w550 w555]
          tunnel: [w550 w552] -> w518
          frame False {
          }
          frame True {
            n207 = property on="Capture Data" class="Bool (strict)"(error in=w555, "Val(Sgnl)"=FALSE ("Value (Signaling)")) -> (error out=w553:errorcluster)  [unwired: 1 in, 1 out]
            n208 = property on="Capture Data" class="Bool (strict)"(error in=w553, "DisabledEnum"=T38."Enabled" ("Disabled")) -> (error out=w552:errorcluster)  [unwired: 1 in, 1 out]
          }
        }
        n209 = Bundle By Name(cluster=T37 {"Run Prog"=FALSE, "Done Stop"=FALSE, "Load Profile"=FALSE, "Save Profile"=FALSE, "Repeat Execution:"=0, "Start Programmer"=FALSE, "Stop Programmer"=FALSE} ("User Selections"), "Done Stop"="Done Stop", "Load Profile"="Load Profile", "Save Profile"="Save Profile", "Repeat Execution:"="Repeat Execution:", "Run Prog"="Run Programmer", "Start Programmer"=w519, "Stop Programmer"=w513) -> (w516:T37)
        n210 = And(x=w513, y="Done Stop") -> (x .and. y?=w512:bool)
        n211 = case shown="True" w512 {
          tunnel: w518 -> [w537 w540]
          tunnel: [w537 w543] -> w517
          tunnel: w516 -> [w536 w542]
          tunnel: [w536 w541] -> w515
          frame False {
          }
          frame True {
            w538 = FALSE ("Run Prog")
            n212 = property on="Run Prog" class="Bool (strict)"(error in=w540, "Value"=w538) -> (error out=w539:errorcluster)  [unwired: 1 in, 1 out]
            n213 = Bundle By Name(cluster=w542, "Run Prog"=w538) -> (w541:T37)
            n214 = property on="Master RUN" class="Bool (strict)"(error in=w539, "Val(Sgnl)"=w538) -> (error out=w543:errorcluster)  [unwired: 1 in, 1 out]
          }
        }
        n215 = call "HXG2programmerFGV.vi"("Programmer Ctrl"=HXG2programmer."Write Selec", "error in (no error)"=w517, "User Selections In"=w515) -> ("error out"=w533:errorcluster)  [unwired: 4 in, 4 out]
      }
      event "CoilData Tabs": Value Change {
        n216 = event-data() -> ()  [unwired: 1 in, 1 out]
        n217 = Unbundle By Name("General_Tube data") -> ("Tube OD"=w565:dbl, "Tube thickness"=w564:dbl)
        n218 = Get Date/Time In Seconds() -> (seconds since 1Jan1904=w568:timestamp)
        n219 = expression code="x*2"(w564) -> (w571:dbl)
        n220 = Get Date/Time String(seconds (now)=w568) -> (date string=w562:string)  [unwired: 2 in, 1 out]
        n221 = Subtract(x=w565, y=w571) -> (x-y=w561:dbl)
        n222 = Bundle By Name(cluster="General_Tube data", "Date"=w562, "Tube ID"=w561, "Tested by"="C. Herrera") -> (w560:T19)
        n223 = call "HXG2_CoilData.vi"("error in (no error)"=w567, "Fin Data"="Fin Data", "General_Tube data"=w560) -> ("error out"=w559:errorcluster, "String Data"=w557:string[])  [unwired: 7 in]
        n224 = property on="General_Tube data" class="Clust (strict)"(error in=w559, "Value"=w560) -> (error out=w558:errorcluster)  [unwired: 1 in, 1 out]
        n225 = call "HXG2_CoilDataFGV.vi"("FGVctrl"=enum16{"Write", "Pass"}."Write", "error in (no error)"=w558, "String Data"=w557) -> ("error out"=w570:errorcluster)  [unwired: 6 in, 2 out]
      }
    }
    n226 = call "HXG2-Error_Module.vi"("error in (no error)"=w53) -> ("error out"=w54:errorcluster)  [unwired: 9 in, 1 out]
    "Event" <- w57
  }
  n227 = while {
    shift-right: [w606] -> _
    shift-left: _ -> [w607]
    shift-right: [w604] -> _
    shift-left: _ -> [w605]
    shift-right: [w602] -> _
    shift-left: _ -> [w603]
    shift-right: [w600] -> _
    shift-left: _ -> [w601]
    shift-right: [w597] -> _
    shift-left: _ -> [w598]
    shift-right: [w596] -> _
    shift-left: _ -> [w595]
    shift-right: [w594] -> _
    shift-left: _ -> [w593]
    shift-right: [w592] -> _
    shift-left: _ -> [w591]
    shift-right: [w590] -> _
    shift-left: _ -> [w589]
    shift-right: [w579] -> w4
    shift-left: w27 -> [w585]
    shift-right: [w582] -> w10
    shift-left: w26 -> [w586]
    tunnel: w22 -> [w578]
    tunnel: w12 -> [w577]
    shift-right: [w574] -> _
    shift-left: refnum<vi> refnum ("Table") -> [w575]
    shift-right: [w572] -> _
    shift-left: FALSE ("MAIN") -> [w573]
    i -> [w587]
    stop <- w588 stop-if-true
    n228 = Dequeue Element(queue=w586, timeout in ms (-1)=100, error in (no error)=w585) -> (queue out=w583:refnum<queue>, element=w581:T1, error out=w584:errorcluster)  [unwired: 1 out]
    "Main Ctrl" <- w581
    n229 = Wait (ms)(milliseconds to wait=u32 100 ("millisecond multiple")) -> ()  [unwired: 1 out]
    n230 = case shown="\"Print\"" w581 {
      tunnel: w584 -> [w658 w705 w800 w840 w862 w900 w965 w1032 w1116 w1170 w1215 w1245]
      tunnel: [w668 w719 w783 w825 w867 w907 w950 w1014 w1105 w1161 w1212 w1238] -> w580
      tunnel: w607 -> [w684 w753 _ w834 w878 w928 w970 w1079 w1122 w1177 w1225 w1259]
      tunnel: [w684 w753 w797 w834 w878 w928 w970 w1079 w1122 w1177 w1225 w1259] -> w606
      tunnel: w605 -> [w683 w752 _ w833 w873 w923 w961 w988 w1114 w1169 w1224 w1258]
      tunnel: [w683 w752 w796 w833 w873 w923 w961 w988 w1114 w1169 w1224 w1258] -> w604
      tunnel: w603 -> [w682 w751 w801 w841 w872 w919 w962 w981 w1115 w1168 w1223 w1257]
      tunnel: [w682 w751 w801 w817 w872 w918 w962 w981 w1115 w1168 w1223 w1257] -> w602
      tunnel: w601 -> [w681 w750 _ w842 w877 w927 w934 w1091 w1121 w1176 w1222 w1256]
      tunnel: [w681 w750 w762 w842 w877 w927 w934 w1091 w1121 w1176 w1222 w1256] -> w600
      tunnel: w598 -> [w680 w749 w795 _ w876 w926 w969 w1090 w1120 w1175 w1221 w1255]
      tunnel: [w680 w749 w795 w827 w876 w926 w969 w1090 w1120 w1175 w1221 w1255] -> w597
      tunnel: [w679 w748 w794 w826 w875 w925 w960 w1027 w1119 w1174 w1220 w1254] -> w596
      tunnel: w595 -> [w679 w748 w794 w806 w875 w925 w960 w1027 w1119 w1174 w1220 w1254]
      tunnel: [w678 w747 w774 w831 w869 w914 w963 w1089 w1110 w1157 w1219 w1247] -> w594
      tunnel: w593 -> [w678 w747 _ w831 w869 w914 w963 w1089 w1110 w1157 w1219 w1247]
      tunnel: [w677 w746 w789 w830 w871 w924 w968 w1088 w1118 w1173 w1218 w1240] -> w592
      tunnel: w591 -> [w677 w746 _ w830 w871 w924 w968 w1088 w1118 w1173 w1218 w1240]
      tunnel: [w676 w745 w792 w829 w868 w915 w967 w1087 w1117 w1172 w1217 w1253] -> w590
      tunnel: w589 -> [w676 w745 w792 w829 w870 w915 w967 w1087 w1117 w1172 w1217 w1253]
      tunnel: [FALSE FALSE FALSE FALSE FALSE FALSE FALSE FALSE FALSE FALSE FALSE TRUE] -> w588
      tunnel: w583 -> [w656 w717 w781 w822 w865 w904 w948 w1010 w1103 w1159 w1209 w1239]
      tunnel: [w666 w718 w782 w821 w863 w903 w947 w1013 w1104 w1160 w1210 w1239] -> w582
      tunnel: w578 -> [w655 _ _ _ _ _ _ _ _ _ _ _]
      tunnel: w577 -> [w652 _ _ _ _ _ _ _ _ _ _ _]
      tunnel: w575 -> [_ w697 w763 w803 w852 w901 w930 w977 w1093 w1131 w1205 w1233]
      tunnel: [w609 w696 w763 w803 w852 w901 w930 w977 w1093 w1131 w1205 w1233] -> w574
      tunnel: w573 -> [w608 w685 w761 w802 w851 w888 w929 w976 w1092 w1130 w1204 w1232]
      tunnel: [w608 w685 w760 w802 w851 w888 w929 w976 w1092 w1130 w1204 w1232] -> w572
      frame "Initialize", Default {
        w627 = FALSE ("AF PID")
        w631 = 0.0 ("Air FLOW %")
        # "Scheduler Table"
        # "All Strings for \nTDMS columns"
        # "Initialize graph scales and labels"
        # "Initialize Keith's programmer"
        n231 = call "HXG2-Error_Module.vi"("user event out"=w652, "Command (Handle Errors)"=HXG2-Error_Module."Initialize", "error in (no error)"=w658, "DAQ Q"=w655, "Main Q"=w656) -> ("error out"=w646:errorcluster)  [unwired: 5 in, 1 out]
        n232 = Bundle By Name(cluster=T7 {"Liq FLOW %"=0.0, "Liq TEMP % "=0.0, "Mdot lbm/hr"=0.0, "TLiq °F"=40.0} ("Value (Signaling)"), "Liq FLOW %"=0.0 ("Air FLOW %"), "Liq TEMP %"=50.0 ("Air FLOW %"), "Mdot lbm/hr"=0.0 ("Air FLOW %"), "TLiq °F"=70.0 ("Air FLOW %")) -> (w621:T7)
        n233 = Bundle By Name(cluster=T8 {"Air FLOW %"=0.0, "Air TEMP % "=0.0, "CFMs"=0.0, "Tair  °F"=0.0} ("Value (Signaling)"), "Air FLOW %"=w631, "Air TEMP %"=50.0 ("Air FLOW %"), "CFMs"=w631, "Tair  °F"=70.0 ("Air FLOW %")) -> (w633:T8)
        n234 = property on="CoilData Tabs" class="TabCtl (strict)"(error in=w646, "Val(Sgnl)"=enum32{"General Data", "Fin Data"}."General Data" ("Value (Signaling)")) -> (error out=w645:errorcluster)  [unwired: 1 in, 1 out]
        n235 = call "Programmer.vi"("Action"=Programmer_Execution_States."Initialize", "error in (no error)"=w645) -> ("error out"=w674:errorcluster)  [unwired: 6 in, 7 out]
        n236 = call "HXG2_GetAllNamesTDMS.vi"("error in (no error)"=w674, "Control"=enum16{"Initialize", "Pass"}."Initialize") -> ("error out"=w637:errorcluster)  [unwired: 8 in, 9 out]
        n237 = property on="Reset PIDs" class="Clust (strict)"(error in=w637) -> (error out=w635:errorcluster, "Controls[]"=w636:refnum<vi>[])  [unwired: 1 in, 1 out]
        n238 = control-ref of="AF PID"() -> (w643:refnum<vi>)
        n239 = control-ref of="AT PID"() -> (w642:refnum<vi>)
        n240 = control-ref of="LF PID"() -> (w641:refnum<vi>)
        n241 = control-ref of="LT PID"() -> (w640:refnum<vi>)
        n242 = property on="Air Cluster" class="Clust (strict)"(error in=w635, "Val(Sgnl)"=w633) -> (error out=w634:errorcluster)  [unwired: 1 in, 1 out]
        n243 = Bundle By Name(cluster=T42 {"AF PID ON"=refnum, "AT PID ON"=refnum, "LT PID ON"=refnum, "LF PID ON"=refnum, "Reset Ctrls"=[]} ("PID Ref cluster"), "AF PID ON"=w643, "AT PID ON"=w642, "LT PID ON"=w641, "LF PID ON"=w640, "Reset Ctrls"=w636) -> (w639:T42)
        n244 = Bundle By Name(cluster=T33 {"AF PID"=FALSE, "AT PID"=FALSE, "LF PID"=FALSE, "LT PID"=FALSE} ("PIDon-off In"), "AF PID"=w627, "AT PID"=w627, "LF PID"=w627, "LT PID"=w627) -> (w626:T33)
        n245 = call "HXG2pidFGV_gainscheduling.vi"("PID Ref cluster"=w639, "error in (no error)"=w634, "PIDfgvCtrl"=HXG2pid."Write PID Refs") -> ("error out"=w638:errorcluster)  [unwired: 8 in, 8 out]
        n246 = call "HXG2pidFGV_gainscheduling.vi"("PIDon-off In"=w626, "error in (no error)"=w638, "PIDfgvCtrl"=HXG2pid."Write PID On-Off") -> ("error out"=w625:errorcluster)  [unwired: 8 in, 8 out]
        n247 = control-ref of="Programmer"() -> (w664:refnum<vi>)
        n248 = control-ref of="Capture Data"() -> (w662:refnum<vi>)
        n249 = control-ref of="Run Prog"() -> (w649:refnum<vi>)
        n250 = control-ref of="Duration Ctrl"() -> (w661:refnum<vi>)
        n251 = control-ref of="Table"() -> (w663:refnum<vi>)
        n252 = property on="Liq Cluster" class="Clust (strict)"(error in=w625, "Val(Sgnl)"=w621) -> (error out=w624:errorcluster)  [unwired: 1 in, 1 out]
        n253 = Bundle By Name(cluster=T43 {"Prog. Indicator"=refnum, "Table"=refnum, "Save Button"=refnum, "Duration Ctrl"=refnum, "Run Prog"=refnum} ("Prog Refs"), "Prog. Indicator"=w664, "Table"=w663, "Save Button"=w662, "Duration Ctrl"=w661, "Run Prog"=w649) -> (w651:T43)
        n254 = control-ref of="Table"() -> (w609:refnum<vi>)
        n255 = call "HXG2programmerFGV.vi"("References in"=w651, "Programmer Ctrl"=HXG2programmer."Write Refs", "error in (no error)"=w624) -> ("error out"=w616:errorcluster)  [unwired: 4 in, 4 out]
        n256 = call "HXG2_PlotScalesSaveFGV.vi"(7:HXG2_GraphSelections."Load From File", "error in (no error)"=w616) -> ("error out"=w613:errorcluster, "Plot Selection Out"=w611:u16[], "Plot Axis Out"=w610:u32[])  [unwired: 5 in, 2 out]
        n257 = property on="Plot Selection" class="Arr (strict)"(error in=w613, "Val(Sgnl)"=w611) -> (error out=w614:errorcluster)  [unwired: 1 in, 1 out]
        n258 = property on="Plot Axis" class="Arr (strict)"(error in=w614, "Val(Sgnl)"=w610) -> (error out=w612:errorcluster)  [unwired: 1 in, 1 out]
        n259 = control-ref of="Air EN"() -> (w672:refnum<vi>)
        n260 = control-ref of="LIQ EN"() -> (w673:refnum<vi>)
        n261 = call "HXG2enableFGV.vi"("LIQ EN"=w673, "ENABLE Ctrl"=HXG2enable."Write Refs" ("ENABLE"), "error in (no error)"=w612, "Air EN"=w672) -> ("error out"=w670:errorcluster)  [unwired: 5 in, 2 out]
        n262 = property on="Apply Scales" class="Bool (strict)"(error in=w670, "Val(Sgnl)"=TRUE ("Value (Signaling)")) -> (error out=w654:errorcluster)  [unwired: 1 in, 1 out]
        n263 = Enqueue Element(queue=w656, element=HXG2_MainStateCtrl."Initialize UI" ("Main State Ctrl"), timeout in ms (-1)=200, error in (no error)=w654) -> (queue out=w666:refnum<queue>, error out=w668:errorcluster)  [unwired: 1 out]
      }
      frame "Initialize UI" {
        w707 = TRUE ("Blinking")
        # "Initialize Table"
        # "Reinitialize colors\n in table"
        # "Start blinking on HX\nID to remind to update"
        # "Initialize the table and UI\nselections for programmer"
        n264 = control-ref of="1\""() -> (w722:refnum<vi>)
        n265 = control-ref of="1.25\""() -> (w721:refnum<vi>)
        n266 = control-ref of="1.5\""() -> (w720:refnum<vi>)
        n267 = control-ref of="Sensor"() -> (w715:refnum<vi>)
        n268 = control-ref of="LiqIn 1 °F"() -> (w744:refnum<vi>)
        n269 = control-ref of="LiqIn 2 °F"() -> (w743:refnum<vi>)
        n270 = control-ref of="LiqOut 1 °F"() -> (w742:refnum<vi>)
        n271 = control-ref of="LiqOut 2 °F"() -> (w741:refnum<vi>)
        n272 = control-ref of="AirIn 1 °F"() -> (w740:refnum<vi>)
        n273 = control-ref of="AirIn 2 °F"() -> (w739:refnum<vi>)
        n274 = control-ref of="AirIn 3 °F"() -> (w738:refnum<vi>)
        n275 = control-ref of="AirIn 4 °F"() -> (w737:refnum<vi>)
        n276 = control-ref of="AirOut 1 °F"() -> (w736:refnum<vi>)
        n277 = control-ref of="AirOut 2 °F"() -> (w735:refnum<vi>)
        n278 = control-ref of="AirOut 3 °F"() -> (w734:refnum<vi>)
        n279 = control-ref of="AirOut 4 °F"() -> (w733:refnum<vi>)
        n280 = control-ref of="AirOut 5 °F"() -> (w732:refnum<vi>)
        n281 = control-ref of="AirOut 6 °F"() -> (w731:refnum<vi>)
        n282 = control-ref of="AirOut 7 °F"() -> (w730:refnum<vi>)
        n283 = control-ref of="AirOut 8 °F"() -> (w729:refnum<vi>)
        n284 = control-ref of="0.75\""() -> (w723:refnum<vi>)
        n285 = property on="HX ID" class="Str"(error in=w705, "Blinking"=w707) -> (error out=w708:errorcluster, "Caption"=w706:refnum<vi>)  [unwired: 1 in, 1 out]
        n286 = control-ref of="Fan TR"() -> (w693:refnum<vi>)
        n287 = control-ref of="Fan TL"() -> (w692:refnum<vi>)
        n288 = control-ref of="Fan BR"() -> (w691:refnum<vi>)
        n289 = control-ref of="Fan BL"() -> (w690:refnum<vi>)
        n290 = Build Array(w744, w743, w742, w741, w740, w739, w738, w737, w736, w735, w734, w733, w732, w731, w730, w729, w723, w722, w721, w720, w715) -> (w726:refnum<vi>[])
        n291 = property class="Txt"(reference=w706, error in=w708, "Visible"=w707) -> (error out=w688:errorcluster)  [unwired: 1 out]
        n292 = control-ref of="Air Cluster"() -> (w728:refnum<vi>)
        n293 = control-ref of="Gly Cluster"() -> (w727:refnum<vi>)
        n294 = Build Array(w693, w692, w691, w690) -> (w689:refnum<vi>[])
        n295 = for {
          tunnel: w689 -> [w757] mode=indexing
          shift-right: [w755] -> w687
          shift-left: w688 -> [w756]
          tunnel: FALSE -> [w754]
          n296 = property class="Bool (strict)"(reference=w757, error in=w756, "Val(Sgnl)"=w754) -> (error out=w755:errorcluster)  [unwired: 1 out]
        }
        n297 = Build Array(w728, w727) -> (w725:refnum<vi>[])
        n298 = call "HXG2_LOAD Config File Values.vi"("error in"=w687, "All Ctrls Refs"=w725, "All Bool Refs"=w726) -> ("error out"=w701:errorcluster, "PID Gains Out"=w700:T12)  [unwired: 7 in]
        n299 = property on="PID Setup Array" class="Arr (strict)"(error in=w701, "Value"=w700) -> (error out=w699:errorcluster)  [unwired: 1 in, 1 out]
        n300 = property class="Tbl (strict)"(reference=w697, error in=w699, "Active Cell"=T45 {"Row"=-2, "Column"=-2} ("Active Cell:Active Cell"), "Cell BG Color"=u32 16777215 ("y")) -> (reference out=w696:refnum<vi>, error out=w698:errorcluster)
        n301 = property on="x-axis length (min)" class="DigNum (strict)"(error in=w698, "Val(Sgnl)"=1.0 ("Value (Signaling)")) -> (error out=w711:errorcluster)  [unwired: 1 in, 1 out]
        n302 = call "HXG2_GroupInitialize.vi"("Profile Name"="StartProf.prof", "error in"=w711) -> ("error out"=w710:errorcluster)  [unwired: 9 in]
        n303 = property on="Clear Alarms" class="Bool (strict)"(error in=w710, "Value"=FALSE ("Clear Alarms")) -> (error out=w704:errorcluster)  [unwired: 1 in, 1 out]
        n304 = property on="x-axis length (min)" class="DigNum (strict)"(error in=w704, "Val(Sgnl)"=1.0 ("Value (Signaling)")) -> (error out=w703:errorcluster)  [unwired: 1 in, 1 out]
        n305 = Enqueue Element(queue=w717, element=HXG2_MainStateCtrl."DAQ" ("Main State Ctrl"), timeout in ms (-1)=200, error in (no error)=w703) -> (queue out=w718:refnum<queue>, error out=w719:errorcluster)  [unwired: 1 out]
      }
      frame "DAQ" {
        # "If programmer is running\nsetpoints are passed here\nover riding UI setpoints"
        # "Pass user set values from\nEvent loop above"
        # "Pass data obtained in\nDAQ loop below"
        n306 = call "HXG2DataTransFGV.vi"("DataTransCtrl"=HXG2DataTrans."Pass", "error in (no error)"=w800) -> ("error out"=w788:errorcluster, "DAQ All"=w799:T51)  [unwired: 8 in]
        n307 = Unbundle By Name(w799) -> ("Digital In"=w797:T34, "Analog In"=w796:T50, "Excel/Elapsed t"=w762:dbl[])
        n308 = call "HXG2programmerFGV.vi"("Programmer Ctrl"=HXG2programmer."Pass All", "error in (no error)"=w788) -> ("error out"=w785:errorcluster, "User Selections Out"=w787:T37)  [unwired: 5 in, 3 out]
        n309 = Unbundle By Name(w787) -> ("Run Prog"=w776:bool)
        n310 = call "HXG2air-glyClusterFGV.vi"("AirGlyCtrl"=HXG2airglyCluster."Pass", "error in (no error)"=w785) -> ("error out"=w778:errorcluster, "AIR-GLY Cluster"=w775:T52)  [unwired: 8 in]
        n311 = control-ref of="Air Cluster"() -> (w767:refnum<vi>)
        n312 = control-ref of="Gly Cluster"() -> (w768:refnum<vi>)
        n313 = call "HXG2_PassSetPoints.vi"("Run Programmer"=w776, "error in (no error)"=w778, "Air Cluster Ref"=w767, "Gly Cluster Ref"=w768, "AIR-GLY Cluster In"=w775) -> ("error out"=w777:errorcluster, "Setpoints"=w769:T53, "AIR-GLY Cluster Out"=w774:T52)  [unwired: 4 in]
        n314 = Unbundle By Name(w769) -> ("Airflow (CFM)"=→"CFM SP":dbl, "Air Temp (°F)"=→"Tair SP °F":dbl, "Glycol Flow (lbm/hr)"=→"Liq SP lbm/hr":dbl, "Glycol Temp(°F)"=→"Tliq SP °F":dbl)
        n315 = call "HXG2pidFGV_gainscheduling.vi"("error in (no error)"=w777, "PIDfgvCtrl"=HXG2pid."Pass") -> ("AirCool Cascade Out"=w758:T47, "LiqHeat Cascade Out"=w759:T48, "PID Resets Out"=w765:T14, "PIDon-off"=w790:T33, "PID Gains Out"=w764:T12, "error out"=w779:errorcluster)  [unwired: 9 in, 3 out]
        n316 = Bundle By Name(cluster=T46 {"PIDon-off "={"AF PID"=FALSE, "AT PID"=FALSE, "LF PID"=FALSE, "LT PID"=FALSE}, "PID"=[], "Reset PIDs"={"AF"=FALSE, "AC"=FALSE, "AH"=FALSE, "LF"=FALSE, "LC"=FALSE, "LH"=FALSE}, "AirCool Cascade"={"PID gains"={"proportional gain (Kc)"=0.0, "integral time (Ti, min)"=0.0, "derivative time (Td, min)"=0.0}, "output range"={"output high"=0.0, "output low"=0.0}}, "LiqHeat Cascade"={"PID gains"={"proportional gain (Kc)"=0.0, "integral time (Ti, min)"=0.0, "derivative time (Td, min)"=0.0}, "output range"={"output high"=0.0, "output low"=0.0}}} ("PID Cluster"), "Reset PIDs"=w765, "PIDon-off"=w790, "PID"=w764, "LiqHeat Cascade"=w759, "AirCool Cascade"=w758) -> (w789:T46)
        n317 = Enqueue Element(queue=w781, element=HXG2_MainStateCtrl."Process" ("Main State Ctrl"), error in (no error)=w779) -> (queue out=w782:refnum<queue>, error out=w783:errorcluster)  [unwired: 1 in, 1 out]
        n318 = Not(x=w761) -> (.not. x?=w760:bool)
        "MAIN" <- w760
      }
      frame "Process" {
        # "Pass Boolean selections\nfrom Event loop above"
        # "RunSS & React to alarms"
        # "Generate\nAlarms"
        # "Control Comp\nContactor"
        n319 = call "HXG2boolselcFGV.vi"("BoolselecFGV"=HXG2boolselec."Pass", "error in (no error)"=w840) -> ("error out"=w839:errorcluster, "BoolSelecOut"=w837:T29)  [unwired: 8 in]
        n320 = call "HXG2_Data Process.vi"("error in"=w839, "Analog DATA In"=w833, "BoolSelection In"=w837, "Calculated Values"=w841) -> ("error out"=w818:errorcluster, "Calculated Values"=w817:T54)  [unwired: 6 in]
        n321 = Unbundle By Name(w817) -> ("Means.Liq In Avg"=w816:dbl, "Means.Liq Out Avg"=w815:dbl, "Liq.Liq Cp (Btu/lb)"=w814:dbl, "Liq.Fltrd Mdot (lbm/hr)"=w813:dbl)
        n322 = Build Array("Repeatability (% of flow)", "Accuracy (%of flow)") -> (w809:dbl[])
        n323 = call "HXG2_PowerUncert.vi"("Tout Liq (°F)"=w815, "Cp (BTU/lbm °F)"=w814, "Mass Flow (lbm/hr)"=w813, "Inlet Temp Uncert (°F)"="Inlet  Uncert (°F)", "Outlet Temp Uncert (°F)"="Outlet  Uncert (°F)", "error in (no error)"=w818, "Tin Liq (°F)"=w816, "% of rate specs"=w809) -> ("Uncertainty Calcs"=→"Liquid Power Uncertainty":T17, "error out"=w805:errorcluster)  [unwired: 10 in]
        n324 = control-ref of="Clear Alarms"() -> (w804:refnum<vi>)
        n325 = call "Programmer.vi"("Action"=Programmer_Execution_States."Register Data", "ANALOG In"=w833, "error in (no error)"=w805, "Calc Values In"=w817) -> ("error out"=w836:errorcluster)  [unwired: 4 in, 7 out]
        n326 = call "HXG2_CompressorLimits.vi"("error in (no error)"=w836, "Analog In"=w833, "Digital In"=w834) -> ("error out"=w835:errorcluster, "Comp Contactor ON?"=w827:bool)  [unwired: 7 in]
        n327 = call "HXG2_Alarm Parser.vi"("Clear Alarms Ref"=w804, "error in (no error)"=w835, "Alarm Cluster In"=w806, "Analog In"=w833, "Digital In"=w834) -> ("error out"=w832:errorcluster, "Alarm Cluster"=w826:T3)  [unwired: 5 in]
        n328 = call "HXG2_Write Cooling Htng.vi"("Comp Contactor ON?"=w827, "error in (no error)"=w832, "Alarm Cluster"=w826) -> ("error out"=w824:errorcluster)  [unwired: 8 in]
        n329 = Enqueue Element(queue=w822, element=HXG2_MainStateCtrl."Control" ("Main State Ctrl"), timeout in ms (-1)=30, error in (no error)=w824) -> (queue out=w821:refnum<queue>, error out=w825:errorcluster)  [unwired: 1 out]
      }
      frame "Control" {
        # "Set all PID reset buttons to false"
        # "Pass contribution of each PID term and RESET to F all PID reset buttons"
        n330 = call "HXG2programmerFGV.vi"("Programmer Ctrl"=HXG2programmer."Pass All", "error in (no error)"=w862) -> ("error out"=w849:errorcluster, "User Selections Out"=w850:T37)  [unwired: 5 in, 3 out]
        n331 = Unbundle By Name(w850) -> ("Run Prog"=w847:bool)
        n332 = call "Programmer.vi"("Action"=Programmer_Execution_States."Get Current Step Index", "error in (no error)"=w849) -> ("Defrost?"=w846:bool, "error out"=w848:errorcluster)  [unwired: 6 in, 6 out]
        n333 = Select(t=w846, s=w847, f=FALSE) -> (s? t:f=w844:bool)
        n334 = call "HXG2_PIDs_No-Array.vi"("Calculated Values"=w872, "PID Cluster"=w871, "AIR-LIQ Cluster"=w869, "error in (no error)"=w848, "Analog In"=w873, "PID Ctrls"=w870, "Defrost?"=w844) -> ("PID Ctrls Out"=w868:T41, "error out"=w858:errorcluster)  [unwired: 11 in]
        n335 = call "HXG2pidFGV_gainscheduling.vi"("error in (no error)"=w858, "PIDfgvCtrl"=HXG2pid."Pass") -> ("Reset ON?"=w853:bool, "PID Refs Out"=w856:T42, "error out"=w855:errorcluster)  [unwired: 9 in, 6 out]
        n336 = Unbundle By Name(w856) -> ("Reset Ctrls"=w854:refnum<vi>[])
        n337 = case shown="True" w853 {
          tunnel: [w879 w882] -> w857
          tunnel: w855 -> [w879 w881]
          tunnel: w854 -> [_ w880]
          frame False {
          }
          frame True {
            n338 = for {
              shift-right: [w887] -> w882
              shift-left: w881 -> [w886]
              tunnel: w880 -> [w885] mode=indexing
              n339 = To Variant(anything=FALSE) -> (Variant=w883:variant)
              n340 = property class="Ctl"(reference=w885, error in=w886, "Val(Sgnl)"=w883) -> (error out=w887:errorcluster)  [unwired: 1 out]
            }
          }
        }
        n341 = call "HXG2pidFGV_gainscheduling.vi"("error in (no error)"=w857, "PID Ctrls"=w868, "PIDfgvCtrl"=HXG2pid."Write PID Efforts") -> ("error out"=w866:errorcluster)  [unwired: 8 in, 8 out]
        n342 = Enqueue Element(queue=w865, element=HXG2_MainStateCtrl."Write" ("Main State Ctrl"), error in (no error)=w866) -> (queue out=w863:refnum<queue>, error out=w867:errorcluster)  [unwired: 1 in, 1 out]
      }
      frame "Write" {
        n343 = call "HXG2boolselcFGV.vi"("BoolselecFGV"=HXG2boolselec."Pass", "error in (no error)"=w900) -> ("error out"=w898:errorcluster, "BoolSelecOut"=w894:T29)  [unwired: 8 in]
        n344 = Unbundle By Name(w894) -> ("Bool.Fan TR"=w893:bool, "Bool.Fan TL"=w892:bool, "Bool.Fan BR"=w891:bool, "Bool.Fan BL"=w890:bool)
        n345 = Build Array(w893, w892, w891, w890) -> (w889:bool[])
        n346 = Unbundle By Name(w923) -> ("ANALOG.Comp Suct P"=w922:dbl, "TCsComp.CompSuct °F"=w921:dbl)
        n347 = call-poly <vilib>:"DAQmx Write.vi"("task/channels in"=refnum<k21> "HX_Cal_Mixers_Digital", "auto start"=TRUE, "data"=w889, "error in"=w898) -> ("error out"=w897:errorcluster)  [unwired: 9 in, 2 out]
        n348 = call "HXG2_EXP Valves to Superheat Ctrl.vi"("error in (no error)"=w897, "Comp Suct Temp"=w921, "Comp Suct P"=w922) -> ("error out"=w917:errorcluster, "Multiplier"=w916:dbl, "Super Heat (°F)"=w920:dbl)  [unwired: 6 in]
        n349 = Bundle By Name(cluster=w919, "SuperHeat.SuperHeat °F"=w920, "SuperHeat.Multiplier"=w916) -> (w918:T54)
        n350 = call "HXG2_Pre-Write.vi"("error in (no error)"=w917, "EXVs Multiplier"=w916, "PID Ctrls"=w915) -> ("error out"=w913:errorcluster, "Analog Ctrl Out"=w902:dbl[])  [unwired: 7 in]
        n351 = call "HXG2daqFGV.vi"("daqFGV"=HXG2daq."Pass", "error in (no error)"=w913) -> ("error out"=w912:errorcluster, "MAX"=w910:T55)  [unwired: 8 in]
        n352 = Unbundle By Name(w910) -> ("OUT.allANALOG.all ANALOG"=w909:refnum<k21>)
        n353 = call "HXG2_WriteAllCtrl.vi"("All Ctrl Array"=w902, "error in"=w912, "Analog Task"=w909) -> ("error out"=w906:errorcluster)  [unwired: 8 in]
        n354 = Enqueue Element(queue=w904, element=HXG2_MainStateCtrl."Save" ("Main State Ctrl"), error in (no error)=w906) -> (queue out=w903:refnum<queue>, error out=w907:errorcluster)  [unwired: 1 in, 1 out]
      }
      frame "Save" {
        n355 = call "HXG2saveFGV.vi"("saveFGV"=HXG2save."Pass", "error in (no error)"=w965) -> ("error out"=w941:errorcluster, "Full Path"=w952:path, "Saving?"=w932:bool, "tdms file out"=w951:refnum<k34>)  [unwired: 5 in, 1 out]
        n356 = call "HXG2saveTimer.vi"("SaveTimerFGV"=HXG2saveTimer."Check", "error in (no error)"=w941) -> ("error out"=w942:errorcluster, "Dur Done?"=w956:bool, "IntDone?"=w955:bool, "Int Elapsed(s)"=→"Interval Ind":dbl, "Dur Elapsed"=→"Duration Ind":dbl)  [unwired: 5 in]
        n357 = And(x=w932, y=w956) -> (x .and. y?=w943:bool)
        n358 = Path To String(path=w952) -> (string=→"File Name":string)
        n359 = Compound Arithmetic op=AND(w955, w932) -> (w944:bool)
        n360 = call "HXG2_Programmer-Save.vi"("Inteval Show?"=w932, "error In"=w942, "Quit? In"=w943, "Save? In"=w944) -> ("error Out"=w940:errorcluster, "Quit? Out"=w936:bool, "Save? Out"=w937:bool, "Inteval Show?"=w935:bool)  [unwired: 4 in]
        "saving..." <- w937
        n361 = property on="Interval Ind" class="DigNum (strict)"(error in=w940, "Visible"=w935) -> (error out=w939:errorcluster)  [unwired: 1 in, 1 out]
        n362 = Not(x=w936) -> (.not. x?=w933:bool)
        n363 = And(x=w933, y=w932) -> (x .and. y?=w931:bool)
        n364 = property on="Duration Ind" class="DigNum (strict)"(error in=w939, "Visible"=w931) -> (error out=w938:errorcluster)  [unwired: 1 in, 1 out]
        n365 = case shown="True" w936 {
          tunnel: w938 -> [w971 w975]
          tunnel: [w971 w973] -> w957
          frame False {
          }
          frame True {
            w972 = FALSE ("Value (Signaling)")
            n366 = property on="Capture Data" class="Bool (strict)"(error in=w975, "Val(Sgnl)"=w972) -> (error out=w974:errorcluster)  [unwired: 1 in, 1 out]
            n367 = property on="File Name" class="Str"(error in=w974, "Visible"=w972) -> (error out=w973:errorcluster)  [unwired: 1 in, 1 out]
          }
        }
        n368 = call "HXG2_WriteTDMS.vi"("Air-Liq Cluster"=w963, "Save?"=w937, "Calcs"=w962, "Excel/Elapsed t"=w934, "DATA In"=w961, "error in"=w957, "tdms file"=w951, "Test Point"="Test Point") -> ("error out"=w949:errorcluster)  [unwired: 6 in, 1 out]
        n369 = Enqueue Element(queue=w948, element=HXG2_MainStateCtrl."Print" ("Main State Ctrl"), error in (no error)=w949) -> (queue out=w947:refnum<queue>, error out=w950:errorcluster)  [unwired: 1 in, 1 out]
      }
      frame "Print" {
        # "This indicator\nshows if Air is\nhigh or low"
        n370 = Unbundle By Name(w988) -> ("ANALOG.Liq Mdot"=→"Liq Flow lbm/hr":dbl, "ANALOG.Pmp  0-250psia"=→"T° @ f/meter":dbl)
        n371 = Unbundle By Name(w988) -> ("ANALOG.Pmp  0-250psia"=w983:dbl, "ANALOG.Pump dP 0-25"=w978:dbl, "TCsComp.CompSuct °F"=→"Suction Temp":dbl, "TCsComp.CompDisch °F"=→"Discharge Temp":dbl)
        "Pump Pout (psia)" <- w983
        "dP Inlet" <- w978
        "Pump Pressure (150psi max)" <- w983
        n372 = Unbundle By Name(w981) -> ("Liq.Liq mu (lbm/ft sec)"=→"Viscosity (lbm/ft s)":dbl, "Liq.Liq Cp (Btu/lb)"=→"Cp (BTU/lbm °F)":dbl, "Liq.Liq Re"=→"Re Number":dbl, "Air.Min ACFM"=→"Min ACFM" →"Min ACFM 2":dbl, "Air.Max ACFM"=→"Max ACFM" →"Max ACFM 2":dbl, "SuperHeat.SuperHeat °F"=→"Comp\nSuct SH":dbl, "Liq.Liq rho (lbm/ft³)"=→"Calc Rho (lbm/ft³)":dbl)
        n373 = Unbundle By Name(w1079) -> ("All Digital IN.EMOreset"=w1023:bool)
        n374 = Unbundle By Name(w981) -> ("Means.Air Q low"=w1031:bool)
        n375 = Unbundle By Name(w981) -> ("Air.CFM HX"=→"Air Flow ACFM":dbl, "Means.Air In Avg"=→"Air Temp °F":dbl, "Means.Liq In Avg"=→"Liq Temp °F":dbl)
        n376 = Cluster To Array(cluster=w1027) -> (array=w1082:T4[])
        n377 = Or Array Elements(Boolean array=w1082) -> (logical OR=w1025:bool)
        n378 = Compound Arithmetic op=OR(w1025, w1023) -> (w1024:bool)
        n379 = Select(t=w1027, s=w1024, f=T3 {"E-Stop"=FALSE, "Liquid\nLevel"=FALSE, "Pump\nVSD"=FALSE, "Blower\nVSD"=FALSE, "Liquid\nHeater"=FALSE, "Air\nHeater"=FALSE, "Master\nSwitch"=FALSE, "Liquid\nPin"=FALSE, "Comp\nOverLoad"=FALSE, "Comp\nDisch P"=FALSE, "Comp \nDisch T"=FALSE, "HX Flood"=FALSE} ("Alarm Cluster 2")) -> (s? t:f=→"Alarm Cluster":T3)
        n380 = Subtract(x=w983, y=w978) -> (x-y=→"Pump Pin (psia)":dbl)
        n381 = Compound Arithmetic op=AND(w1025, w1023) -> (w1034:bool)
        n382 = Unbundle By Name(w988) -> ("ANALOG.Pmp  0-250psia"=→"Pump Pressure":dbl, "ANALOG.UUT  0-100psid"=→"HX dP":dbl, "ANALOG.UUT 0-50psia"=→"HX Pressure In":dbl, "ANALOG.Liq Mdot"=→"GlyFlow lbm/hr":dbl, "ANALOG.Pmp  0-250psia"=→"LiqRho lb/ft³":dbl)
        n383 = Unbundle By Name(w981) -> ("dT.Air dT °F"=→"dT Air":dbl, "dT.Liq dT °F"=→"dT Liq":dbl)
        n384 = Exclusive Or(1:w1034, 2:w1025) -> (0:w1033:bool)
        n385 = Select(t="Air is Low", s=w1031, f="Air is High") -> (s? t:f=w999:string)
        "%Bal2" <- w999
        n386 = local write "Alarm Set Button"(w1033) -> ()
        n387 = local write "Alarm Set Button"(w1025) -> ()
        n388 = property on="%Bal" class="Str"(error in=w1032, "Value"=w999) -> (error out=w1012:errorcluster)  [unwired: 1 in, 1 out]
        n389 = Unbundle By Name(w988) -> ("ANALOG.Liq in 1"=→"GlyIn 1":dbl, "ANALOG.Liq in 2"=→"GlyIn 2":dbl, "ANALOG.Liq out 1"=→"GlyOut 1":dbl, "ANALOG.Liq out 2"=→"GlyOut 2":dbl, "ANALOG.AIR in 1"=→"AirIn 1":dbl, "ANALOG.AIR in 2"=→"AirIn 2":dbl, "ANALOG.AIR in 3"=→"AirIn 3":dbl, "ANALOG.AIR in 4"=→"AirIn 4":dbl, "ANALOG.AIR out 1"=→"AirOut 1":dbl, "ANALOG.AIR out 2"=→"AirOut 2":dbl, "ANALOG.AIR out 3"=→"AirOut 3":dbl, "ANALOG.AIR out 4"=→"AirOut 4":dbl, "ANALOG.AIR out 5"=→"AirOut 5":dbl, "ANALOG.AIR out 6"=→"AirOut 6":dbl, "ANALOG.AIR out 7"=→"AirOut 7":dbl, "ANALOG.AIR out 8"=→"AirOut 8":dbl, "ANALOG.RH in Temp"=→"UUT °F":dbl, "ANALOG.RH in"=→"UUT %RH":dbl, "ANALOG.Comp Suct P"=→"Comp Suct P psia":dbl, "ANALOG.Pabs nozzle"=→"Baro psia":dbl, "ANALOG.Nozzle dp 0-5"=→"Nozzle dP 5inWC":dbl, "ANALOG.RHout Temp"=→"Nozzle °F":dbl, "ANALOG.RH out"=→"Nozzle %RH":dbl, "ANALOG.UUT dp 0-pt1"=→"UUT dP 0-0.1":dbl, "ANALOG.UUT dP 0-1"=→"UUT dP 0-1.0":dbl, "ANALOG.Nozzle dP 0-2.5"=→"Nozzle dP 2.5inWC":dbl)
        n390 = Unbundle By Name(w981) -> ("Means.Liq In Avg"=→"LiqIn Avg °F" →"Tliq  °F":dbl, "Means.Liq Out Avg"=→"LiqOut Avg °F":dbl, "Means.Air In Avg"=→"AirIn Avg °F" →"Tair  °F":dbl, "Means.Air Out Avg"=→"AirOut Avg °F":dbl, "Means.%Energy Bal"=→"% Balance":dbl, "Means.%Energy Bal"=→"% Balance":dbl, "Liq.Liq Cp (Btu/lb)"=→"LiqCp BTU/lb°F":dbl, "Liq.Liq Q (Btu/hr)"=→"Liq q BTU/hr":dbl, "Liq.Liq Q (W)"=→"Liq q W":dbl, "Air.Air Q (Btu/hr)"=→"Air q BTU/hr":dbl, "Air.Air Q (W)"=→"Air q W":dbl, "Air.CFM nozzle"=→"AirFlow SCFM":dbl, "Air.CFM HX"=→"AirFlow ACFM" →"CFM":dbl, "Air.Air Cp (Btu/lb)"=→"AirCp BTU/lb°F":dbl, "Air.Air rho (lbm/ft³)"=→"AirRho lb/ft³":dbl, "Liq.Fltrd Mdot (lbm/hr)"=→"Filtered Mdot lbm/hr":dbl)
        n391 = Unbundle By Name(w988) -> ("ANALOG.TC in 1"=→"UUTIn 1":dbl, "ANALOG.TC in 2"=→"UUTIn 2":dbl, "ANALOG.TC in 3"=→"UUTIn 3":dbl, "ANALOG.TC in 4"=→"UUTIn 4":dbl, "ANALOG.TC in 5"=→"UUTIn 5":dbl, "ANALOG.TC in 6"=→"UUTIn 6":dbl, "ANALOG.TC in 7"=→"UUTIn 7":dbl, "ANALOG.TC in 8"=→"UUTIn 8":dbl)
        n392 = Unbundle By Name(w988) -> ("TCsComp.LiqHtrWell °F"=→"Liq Htr Well":dbl, "ANALOG.TC in 9"=→"UUTIn 9":dbl, "ANALOG.TC in 10"=→"UUTIn 10":dbl, "ANALOG.TC in 11"=→"UUTIn 11":dbl, "ANALOG.TC in 12"=→"UUTIn 12":dbl, "ANALOG.TC in 13"=→"UUTIn 13":dbl, "ANALOG.TC in 14"=→"UUTIn 14":dbl, "ANALOG.TC in 15"=→"UUTIn 15":dbl, "ANALOG.TC in 16"=→"UUTIn 16":dbl)
        n393 = Unbundle By Name(w981) -> ("Means.Air Evap Avg"=→"EvapAvg":dbl, "Means.Air Htr Avg"=→"HtrAvg":dbl)
        n394 = Enqueue Element(queue=w1010, element=HXG2_MainStateCtrl."Graph" ("Main State Ctrl"), error in (no error)=w1012) -> (queue out=w1013:refnum<queue>, error out=w1014:errorcluster)  [unwired: 1 in, 1 out]
        "Alarm Present\nLED" <- "Alarm Set Button"
      }
      frame "Graph" {
        n395 = Unbundle By Name(w1110) -> ("Air Cluster.CFMs"=→"Air flow":dbl, "Air Cluster.Tair  °F"=→"Air Temp":dbl, "Liq Cluster.Mdot lbm/hr"=→"Mass flow":dbl, "Liq Cluster.TLiq °F"=→"Liq Temp":dbl)
        n396 = call "HXG2_AlldataToArray.vi"("error in (no error)"=w1116, "Calculated Values"=w1115, "Analog In"=w1114) -> ("error out"=w1100:errorcluster, "Strings Out"=w1099:string[], "Plot"=w1113:dbl[])  [unwired: 6 in]
        n397 = First Call?() -> (First Call?: T/F=w1098:bool)
        n398 = case shown="True" w1098 {
          tunnel: w1100 -> [w1123 w1126]
          tunnel: w1099 -> [_ w1124]
          tunnel: [w1123 w1127] -> w1096
          frame False {
          }
          frame True {
            n399 = property on="Channels" class="Ring (strict)"(error in=w1126, "Strings []"=w1124) -> (error out=w1125:errorcluster)  [unwired: 1 in, 1 out]
            n400 = property on="Prof 1" class="Ring (strict)"(error in=w1125, "Strings []"=w1124) -> (error out=w1129:errorcluster)  [unwired: 1 in, 1 out]
            n401 = property on="Prof 2" class="Ring (strict)"(error in=w1129, "Strings []"=w1124) -> (error out=w1128:errorcluster)  [unwired: 1 in, 1 out]
            n402 = property on="Prof 3" class="Ring (strict)"(error in=w1128, "Strings []"=w1124) -> (error out=w1127:errorcluster)  [unwired: 1 in, 1 out]
          }
        }
        n403 = call "HXG2_PlotScalesSaveFGV.vi"(7:HXG2_GraphSelections."Out", "error in (no error)"=w1096) -> ("error out"=w1097:errorcluster, "Plot Selection Out"=w1094:u16[])  [unwired: 5 in, 3 out]
        n404 = call "HXG2_SelectDataToPlot.vi"("Plot Selection"=w1094, "error IO"=w1097, "Numeric Array In"=w1113) -> ("error Out"=w1101:errorcluster, "Array of Waveform Out"=→"Waveform Chart Out":waveform(dbl)[])  [unwired: 7 in]
        n405 = Enqueue Element(queue=w1103, element=HXG2_MainStateCtrl."Sequencer" ("Main State Ctrl"), error in (no error)=w1101) -> (queue out=w1104:refnum<queue>, error out=w1105:errorcluster)  [unwired: 1 in, 1 out]
      }
      frame "Sequencer" {
        n406 = control-ref of="Run Programmer"() -> (w1154:refnum<vi>)
        n407 = call "HXG2_SequencerGroup.vi"("error In"=w1170, "Bool Refnum"=w1154, "Calculated Values"=w1168, "Analog In"=w1169) -> ("error out"=w1155:errorcluster, "Programmer State"=w1138:T15, "Running?"=w1144:bool, "Components Stable?"=w1167:bool[], "Current Step"=w1145:i32)  [unwired: 2 in, 1 out]
        "Current Step" <- w1145
        "Programmer State" <- w1138
        "Programmer" <- w1144
        n408 = property on="Test Point" class="DigNum (strict)"(error in=w1155, "Value"=w1145) -> (error out=w1156:errorcluster)  [unwired: 1 in, 1 out]
        n409 = property on="Programmer" class="Bool (strict)"(error in=w1156, "Blinking"=w1144) -> (error out=w1153:errorcluster)  [unwired: 1 in, 1 out]
        n410 = call "HXG2_ProgCntDowns.vi"("FGVctrl"=enum16{"Write", "Pass"}."Pass", "error in (no error)"=w1153) -> ("error out"=w1150:errorcluster, "Exec t (sec)"=→"Timer":dbl)  [unwired: 8 in]
        n411 = property on="Programmer State" class="Enum (strict)"(error in=w1150) -> (error out=w1149:errorcluster, "RingText.Text"=→"Ring Text.Text":string)  [unwired: 1 in, 1 out]
        n412 = property on="Timer" class="DigNum (strict)"(error in=w1149, "Visible"=w1144) -> (error out=w1147:errorcluster)  [unwired: 1 in, 1 out]
        n413 = Array To Cluster(array=w1167) -> (cluster=w1166:T56)
        n414 = property on="Ring Text.Text" class="Str"(error in=w1147, "Visible"=w1144) -> (error out=w1146:errorcluster)  [unwired: 1 in, 1 out]
        n415 = Unbundle(w1166) -> ("Components Stable?[0]"=→"AirFlow Stable":bool, "Components Stable?[1]"=→"AirTemp Stable":bool, "Components Stable?[2]"=→"LiqFlow Stable":bool, "Components Stable?[3]"=→"LiqTemp Stable":bool)
        n416 = case shown="True" w1144 {
          selector: w1144 -> [w1194 w1199]
          tunnel: w1146 -> [w1197 w1203]
          tunnel: [w1197 w1202] -> w1143
          tunnel: w1145 -> [w1195 w1200]
          tunnel: [w1196 w1201] -> w1134
          tunnel: w1131 -> [w1196 w1201]
          tunnel: [w1195 w1198] -> w1133
          tunnel: [w1194 w1199] -> w1132
          frame False {
          }
          frame True {
            n417 = call "HXG2_TableFormattingForActiveTestPoint.vi"("Current Step"=w1200, "error IO"=w1203, "Table Control"=w1201) -> ("error out"=w1202:errorcluster, "Current Step Out"=w1198:i32)  [unwired: 7 in]
          }
        }
        n418 = Equal?(x=Programmer_State."Running" ("Programmer State"), y=w1138) -> (x = y?=w1139:bool)
        n419 = feedback #1() -> (w1137:T15)  [unwired: 1 in]
        n420 = Not Equal?(x=w1137, y=w1138) -> (x != y?=w1136:bool)
        n421 = Compound Arithmetic op=AND(w1136, w1139, w1132) -> (w1135:bool)
        n422 = case shown="True" w1135 {
          tunnel: w1143 -> [w1182 w1192]
          tunnel: [w1181 w1192] -> w1142
          tunnel: w1138 -> [w1183 w1193]
          tunnel: [w1183 w1193] -> w1141
          tunnel: w1134 -> [w1180 _]
          tunnel: w1133 -> [w1178 _]
          frame True {
            # "If step reached stability cell will be green"
            n423 = for {
              N: 11 -> [_]
              tunnel: w1180 -> [w1189]
              shift-right: [w1190] -> w1181
              shift-left: w1182 -> [w1191]
              tunnel: w1178 -> [w1185]
              i -> [w1188]
              n424 = Bundle By Name(cluster=T45 {"Row"=0, "Column"=0} ("Active Cell:Active Cell"), "Row"=w1185, "Column"=w1188) -> (w1187:T45)
              n425 = property class="Tbl (strict)"(reference=w1189, error in=w1191, "Active Cell"=w1187, "Cell BG Color"=u32 11403127) -> (error out=w1190:errorcluster)  [unwired: 1 out]
            }
          }
          frame False {
          }
        }
        n426 = feedback-in #1(w1141) -> ()
        n427 = Enqueue Element(queue=w1159, element=HXG2_MainStateCtrl."ERROR" ("Main State Ctrl"), error in (no error)=w1142) -> (queue out=w1160:refnum<queue>, error out=w1161:errorcluster)  [unwired: 1 in, 1 out]
      }
      frame "ERROR" {
        n428 = Unbundle By Name(w1215) -> ("status"=w1214:bool)
        n429 = case shown="True" w1214 {
          tunnel: [w1227 w1229] -> w1211
          tunnel: [FALSE ("STOP?") TRUE ("STOP?")] -> w1208
          tunnel: w1215 -> [w1227 w1230]
          frame False {
          }
          frame True {
            n430 = property on="stop" class="Bool (strict)"(error in=w1230, "Val(Sgnl)"=TRUE) -> (error out=w1229:errorcluster)  [unwired: 1 in, 1 out]
          }
        }
        n431 = Select(t=HXG2_MainStateCtrl."Exit" ("Main State Ctrl"), s=w1208, f=HXG2_MainStateCtrl."DAQ" ("Main State Ctrl")) -> (s? t:f=w1206:T1)
        n432 = Enqueue Element(queue=w1209, element=w1206, error in (no error)=w1211) -> (queue out=w1210:refnum<queue>, error out=w1212:errorcluster)  [unwired: 1 in, 1 out]
      }
      frame "Exit" {
        w1235 = T9 FALSE ("Value (Signaling)")
        # "STOP AIR AND LIQUID FLOW\nBEFORE STOPPING PROGRAM"
        n433 = disable-structure shown="Disabled" {
          disable-tunnel: w1245 -> [w1261 w1263]
          disable-tunnel: [w1260 w1263] -> w1234
          frame Disabled {
            n434 = call "HXG2programmerFGV.vi"("Programmer Ctrl"=HXG2programmer."Write All", "error in (no error)"=w1261) -> ("error out"=w1260:errorcluster)  [unwired: 5 in, 4 out]
          }
          frame Enabled {
          }
        }
        n435 = property on="Air EN" class="Bool (strict)"(error in=w1234, "Val(Sgnl)"=w1235) -> (error out=w1237:errorcluster)  [unwired: 1 in, 1 out]
        n436 = property on="LIQ EN" class="Bool (strict)"(error in=w1237, "Val(Sgnl)"=w1235) -> (error out=w1236:errorcluster)  [unwired: 1 in, 1 out]
        n437 = call "HXG2boolselcFGV.vi"("BoolselecFGV"=HXG2boolselec."Pass", "error in (no error)"=w1236) -> ("error out"=w1249:errorcluster, "BoolSelecOut"=w1248:T29)  [unwired: 8 in]
        n438 = call "HXG2_SAVE Config File Values.vi"("error in"=w1249, "BoolSelecOut"=w1248, "AIR-GLY Cluster"=w1247) -> ("error out"=w1241:errorcluster)  [unwired: 8 in]
        n439 = call "HXG2saveFGV.vi"("saveFGV"=HXG2save."Kill", "error in (no error)"=w1241) -> ("error out"=w1244:errorcluster)  [unwired: 5 in, 4 out]
        n440 = property on="Capture Data" class="Bool (strict)"(error in=w1244, "Value"=FALSE ("Capture Data")) -> (error out=w1243:errorcluster)  [unwired: 1 in, 1 out]
        n441 = call "HXG2daqFGV.vi"("daqFGV"=HXG2daq."Stop", "error in (no error)"=w1243) -> ("error out"=w1238:errorcluster)  [unwired: 8 in, 1 out]
      }
    }
    n442 = call "HXG2-Error_Module.vi"("error in (no error)"=w580) -> ("error out"=w579:errorcluster)  [unwired: 9 in, 1 out]
    "Main" <- w587
  }
  n443 = while {
    shift-right: [w1275] -> _
    shift-left: _ -> [w1276]
    shift-right: [w1264] -> w7
    shift-left: w32 -> [w1273]
    shift-right: [w1268] -> w6
    shift-left: w22 -> [w1271]
    i -> [w1274]
    stop <- w1267 stop-if-true
    n444 = Dequeue Element(queue=w1271, timeout in ms (-1)=100, error in (no error)=w1273) -> (queue out=w1270:refnum<queue>, element=w1269:T2, error out=w1272:errorcluster)  [unwired: 1 out]
    "DAQ Control" <- w1269
    n445 = Wait (ms)(milliseconds to wait=u32 80 ("millisecond multiple")) -> ()  [unwired: 1 out]
    n446 = case shown="\"DAQ\"" w1269 {
      tunnel: w1276 -> [w1287 w1317 _]
      tunnel: [w1279 w1317 w1325] -> w1275
      tunnel: w1272 -> [w1304 w1314 w1326]
      tunnel: [w1299 w1314 w1323] -> w1265
      tunnel: [FALSE ("status") TRUE ("status") FALSE ("status")] -> w1267
      tunnel: w1270 -> [w1297 w1315 w1321]
      tunnel: [w1296 w1315 w1322] -> w1268
      frame "DAQ" {
        # "Elapsed t"
        # "Excel Time"
        # "Days from 1900-1904"
        # "seconds in a year"
        n447 = Get Date/Time In Seconds() -> (seconds since 1Jan1904=w1279:timestamp)
        n448 = call "HXG2daqFGV.vi"("daqFGV"=HXG2daq."Pass", "error in (no error)"=w1304) -> ("error out"=w1307:errorcluster, "MAX"=w1313:T55)  [unwired: 8 in]
        n449 = To Double Precision Float(number=w1279) -> (double precision float=w1288:dbl)
        n450 = To Double Precision Float(number=w1287) -> (double precision float=w1289:dbl)
        n451 = Unbundle By Name(w1313) -> ("IN.all Digital"=w1302:refnum<k21>, "IN.Freq_Mdot"=w1300:refnum<k21>)
        n452 = Subtract(x=w1288, y=w1289) -> (x-y=w1311:dbl)
        n453 = expression code="x/86400"(w1288) -> (w1293:dbl)
        n454 = expression code="x/60"(w1311) -> (w1291:dbl)
        n455 = expression code="x+1462"(w1293) -> (w1292:dbl)
        n456 = call "HXG2_Digital-IN.vi"("error in (no error)"=w1307, "FreqMdot Task In"=w1300, "DIG IN TASK"=w1302) -> ("error out"=w1306:errorcluster, "Mdot (lbm/hr)"=w1301:dbl, "Digital In"=w1309:T34)  [unwired: 6 in]
        n457 = call "HXG2_Analog-IN_Final.vi"("error in (no error)"=w1306, "ANALOG.Liq Mdot"=w1301, "MAX"=w1313) -> ("error out"=w1305:errorcluster, "ANALOG OUT"=w1308:T50)  [unwired: 7 in]
        n458 = Build Array(w1292, w1291) -> (w1290:dbl[])
        n459 = call "HXG2DataTransFGV.vi"("DataTransCtrl"=HXG2DataTrans."Write", "error in (no error)"=w1305, "Analog In"=w1308, "Digital In"=w1309, "Excel/Elapsed t"=w1290) -> ("error out"=w1298:errorcluster)  [unwired: 5 in, 1 out]
        n460 = feedback #2(TRUE) -> (w1280:bool)
        n461 = feedback #3() -> (w1284:timestamp)  [unwired: 1 in]
        n462 = To Double Precision Float(number=w1284) -> (double precision float=w1283:dbl)
        n463 = expression code="x+1"(w1283) -> (w1281:dbl)
        n464 = Select(t=w1279, s=w1280, f=w1284) -> (s? t:f=w1286:timestamp)
        n465 = feedback-in #3(w1286) -> ()
        n466 = To Double Precision Float(number=w1279) -> (double precision float=w1282:dbl)
        n467 = Enqueue Element(queue=w1297, element=HXG2_DAQLOOPctrl."DAQ" ("DAQ Control"), timeout in ms (-1)=100, error in (no error)=w1298) -> (queue out=w1296:refnum<queue>, error out=w1299:errorcluster)  [unwired: 1 out]
        n468 = Greater Or Equal?(x=w1282, y=w1281) -> (x >= y?=w1278:bool)
        "DAQ" <- w1278
        n469 = feedback-in #2(w1278) -> ()
      }
      frame "Stop" {
      }
      frame "Initialize" {
        # "Initialize all data collection tasks.  All DAQ in loop below"
        # "Write the constants for all the tasks\nbefore the DAQ is initialized"
        n470 = Get Date/Time In Seconds() -> (seconds since 1Jan1904=w1325:timestamp)
        n471 = call "HXG2daqFGV.vi"("daqFGV"=HXG2daq."Write", "error in (no error)"=w1326) -> ("error out"=w1328:errorcluster)  [unwired: 8 in, 1 out]
        n472 = call "HXG2daqFGV.vi"("daqFGV"=HXG2daq."Initialize", "error in (no error)"=w1328) -> ("error out"=w1320:errorcluster)  [unwired: 8 in, 1 out]
        n473 = Enqueue Element(queue=w1321, element=HXG2_DAQLOOPctrl."DAQ" ("DAQ Control"), timeout in ms (-1)=100, error in (no error)=w1320) -> (queue out=w1322:refnum<queue>, error out=w1323:errorcluster)  [unwired: 1 out]
      }
    }
    n474 = call "HXG2-Error_Module.vi"("error in (no error)"=w1265) -> ("error out"=w1264:errorcluster)  [unwired: 9 in, 1 out]
    "daq" <- w1274
  }
  n475 = Merge Errors(w8, w4, w7) -> (w11:errorcluster)
  n476 = Release Queue(queue=w10, error in (no error)=w11) -> (error out=w9:errorcluster)  [unwired: 1 in, 2 out]
  n477 = Release Queue(queue=w6, error in (no error)=w9) -> (error out=w3:errorcluster)  [unwired: 1 in, 2 out]
  n478 = Unregister For Events(event registration refnum=w13, error in=w3) -> (error out=w14:errorcluster)
  n479 = Destroy User Event(user event=w12, error in=w14) -> (error out=w5:errorcluster)
  n480 = call "HXG2-Error_Module.vi"("Command (Handle Errors)"=HXG2-Error_Module."Report", "error in (no error)"=w5) -> ("error out"=w21:errorcluster)  [unwired: 8 in, 1 out]
  n481 = call <vilib>:"General Error Handler.vi"("type of dialog (OK msg:1)"=w39, "error in (no error)"=w21) -> ("error out"=w37:errorcluster)  [unwired: 9 in, 4 out]
  n482 = property on="stop" class="Bool (strict)"(error in=w37, "Value"=FALSE ("stop")) -> (error out=→"error out":errorcluster)  [unwired: 1 in, 1 out]
